vi "Autonomous Independent.vi"() -> ()   [LabVIEW 2011]
doc: "This VI is called when autonomous begins, and will automatically be terminated when autonomous ends. You can carry out timed or sensor driven robot movement independently without needing to return to the caller."
uses:
  AutoDriveType.ctl
  AutonomousType.ctl
  StateMachineType.ctl
  Robot Global Data.vi
  <vilib>/addons/control/pid/pid.llb/PID (DBL).vi
  <vilib>/Rock Robotics/WPI/RobotDrive/WPI_RobotDriveArcadeDrive_Standard(NoSaturation).vi
  BasketType.ctl
  <vilib>/addons/control/pid/NI_PID_pid.lvlib
panel:
  out "LaunchCounter 3":i32
  out "LaunchCounter 2":i32
  out "LaunchCounter":i32
  in  "AutoDrive":T1
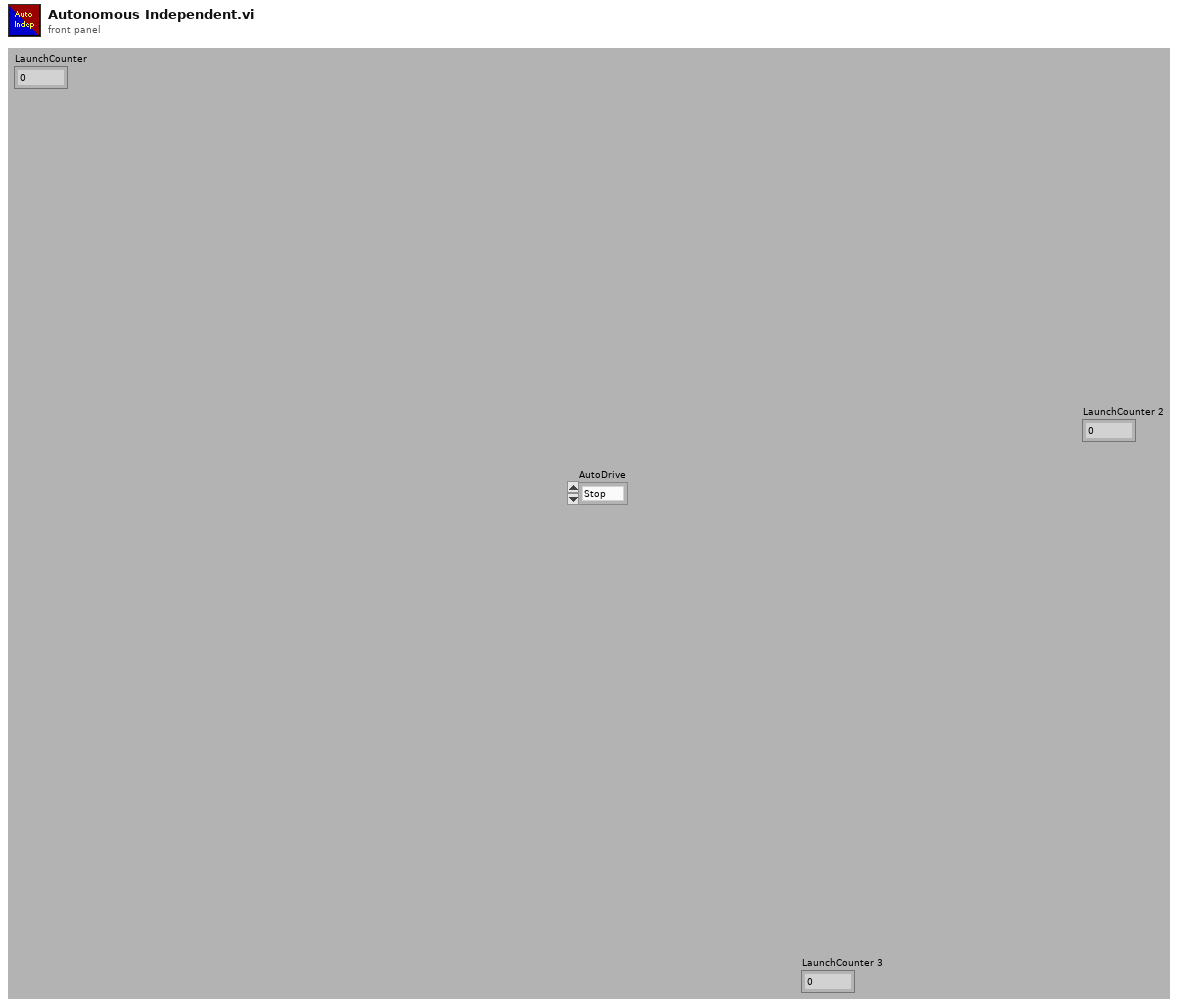
[diagram p1: front panel]
types:
  T1 = typedef "AutoDriveType.ctl" = enum16{"Stop", "DoNothing", "Drive"}
  T2 = typedef "WPI_RobotDriveDevRef.ctl" = cluster{"DevStatus":errorcluster, "Motors[]":T3[], "Square Inputs":bool, "Max Output":dbl, "Isochronous":bool}
  T3 = typedef "WPI_MotorControlDeviceRef.ctl" = cluster{"DeviceStatus":errorcluster, "Type":enum16{"PWM", "CAN"}, "PWM":cluster{"Digital Module":T4, "PWM Channel":T5, "DeadBand":T6}, "CAN":cluster{"Device Number":u8, "Control Mode":T7, "Semaphore":T8, "Max Vout":dbl}, "Invert":bool, "TransformRef":T9, "InvTransformRef":T9}
  T4 = typedef "FPGA_TypedefDigitalModule.ctl" = enum16{"Digital Module 1", "Digital Module 2"}
  T5 = typedef "FPGA_DIOPWMChannel.ctl" = enum8{"PWM 1", "PWM 2", "PWM 3", "PWM 4", "PWM 5", "PWM 6", "PWM 7", "PWM 8", "PWM 9", "PWM 10", "Invalid"}
  T6 = typedef "WPI_PWMDeadband.ctl" = cluster{"Name":string, "maxPositivePwm":i32, "minPositivePwm":i32, "centerPwm":i32, "maxNegativePwm":i32, "minNegativePwm":i32, "angularRange":u16}
  T7 = typedef "WPI_CANJaguar_ControlMode.ctl" = enum8{"Percent VBus", "Current", "Speed", "Position", "Voltage"}
  T8 = typedef "Semaphore RefNum" = refnum<k1>
  T9 = typedef "WPI_PWMTransform_ConPane.ctl" = refnum<vi>
  T10 = typedef "AutonomousType.ctl" = enum16{"Init", "ManualAim", "AutoAim", "Fire", "Drive", "Tip Ramp", "Stop"}
  T11 = typedef "BasketType.ctl" = enum16{"Left", "Bottom", "Right", "Top"}
  T12 = typedef "StateMachineType.ctl" = enum16{"Init", "Idle", "Start", "Do", "Stop"}
  T13 = cluster{"proportional gain (Kc)":dbl, "integral time (Ti, min)":dbl, "derivative time (Td, min)":dbl}
  T14 = cluster{"Position":cluster{"X":dbl, "Y":dbl}, "Distance (ft)":dbl}[]
  T15 = cluster{"Position":cluster{"X":dbl, "Y":dbl}, "Distance (ft)":dbl}
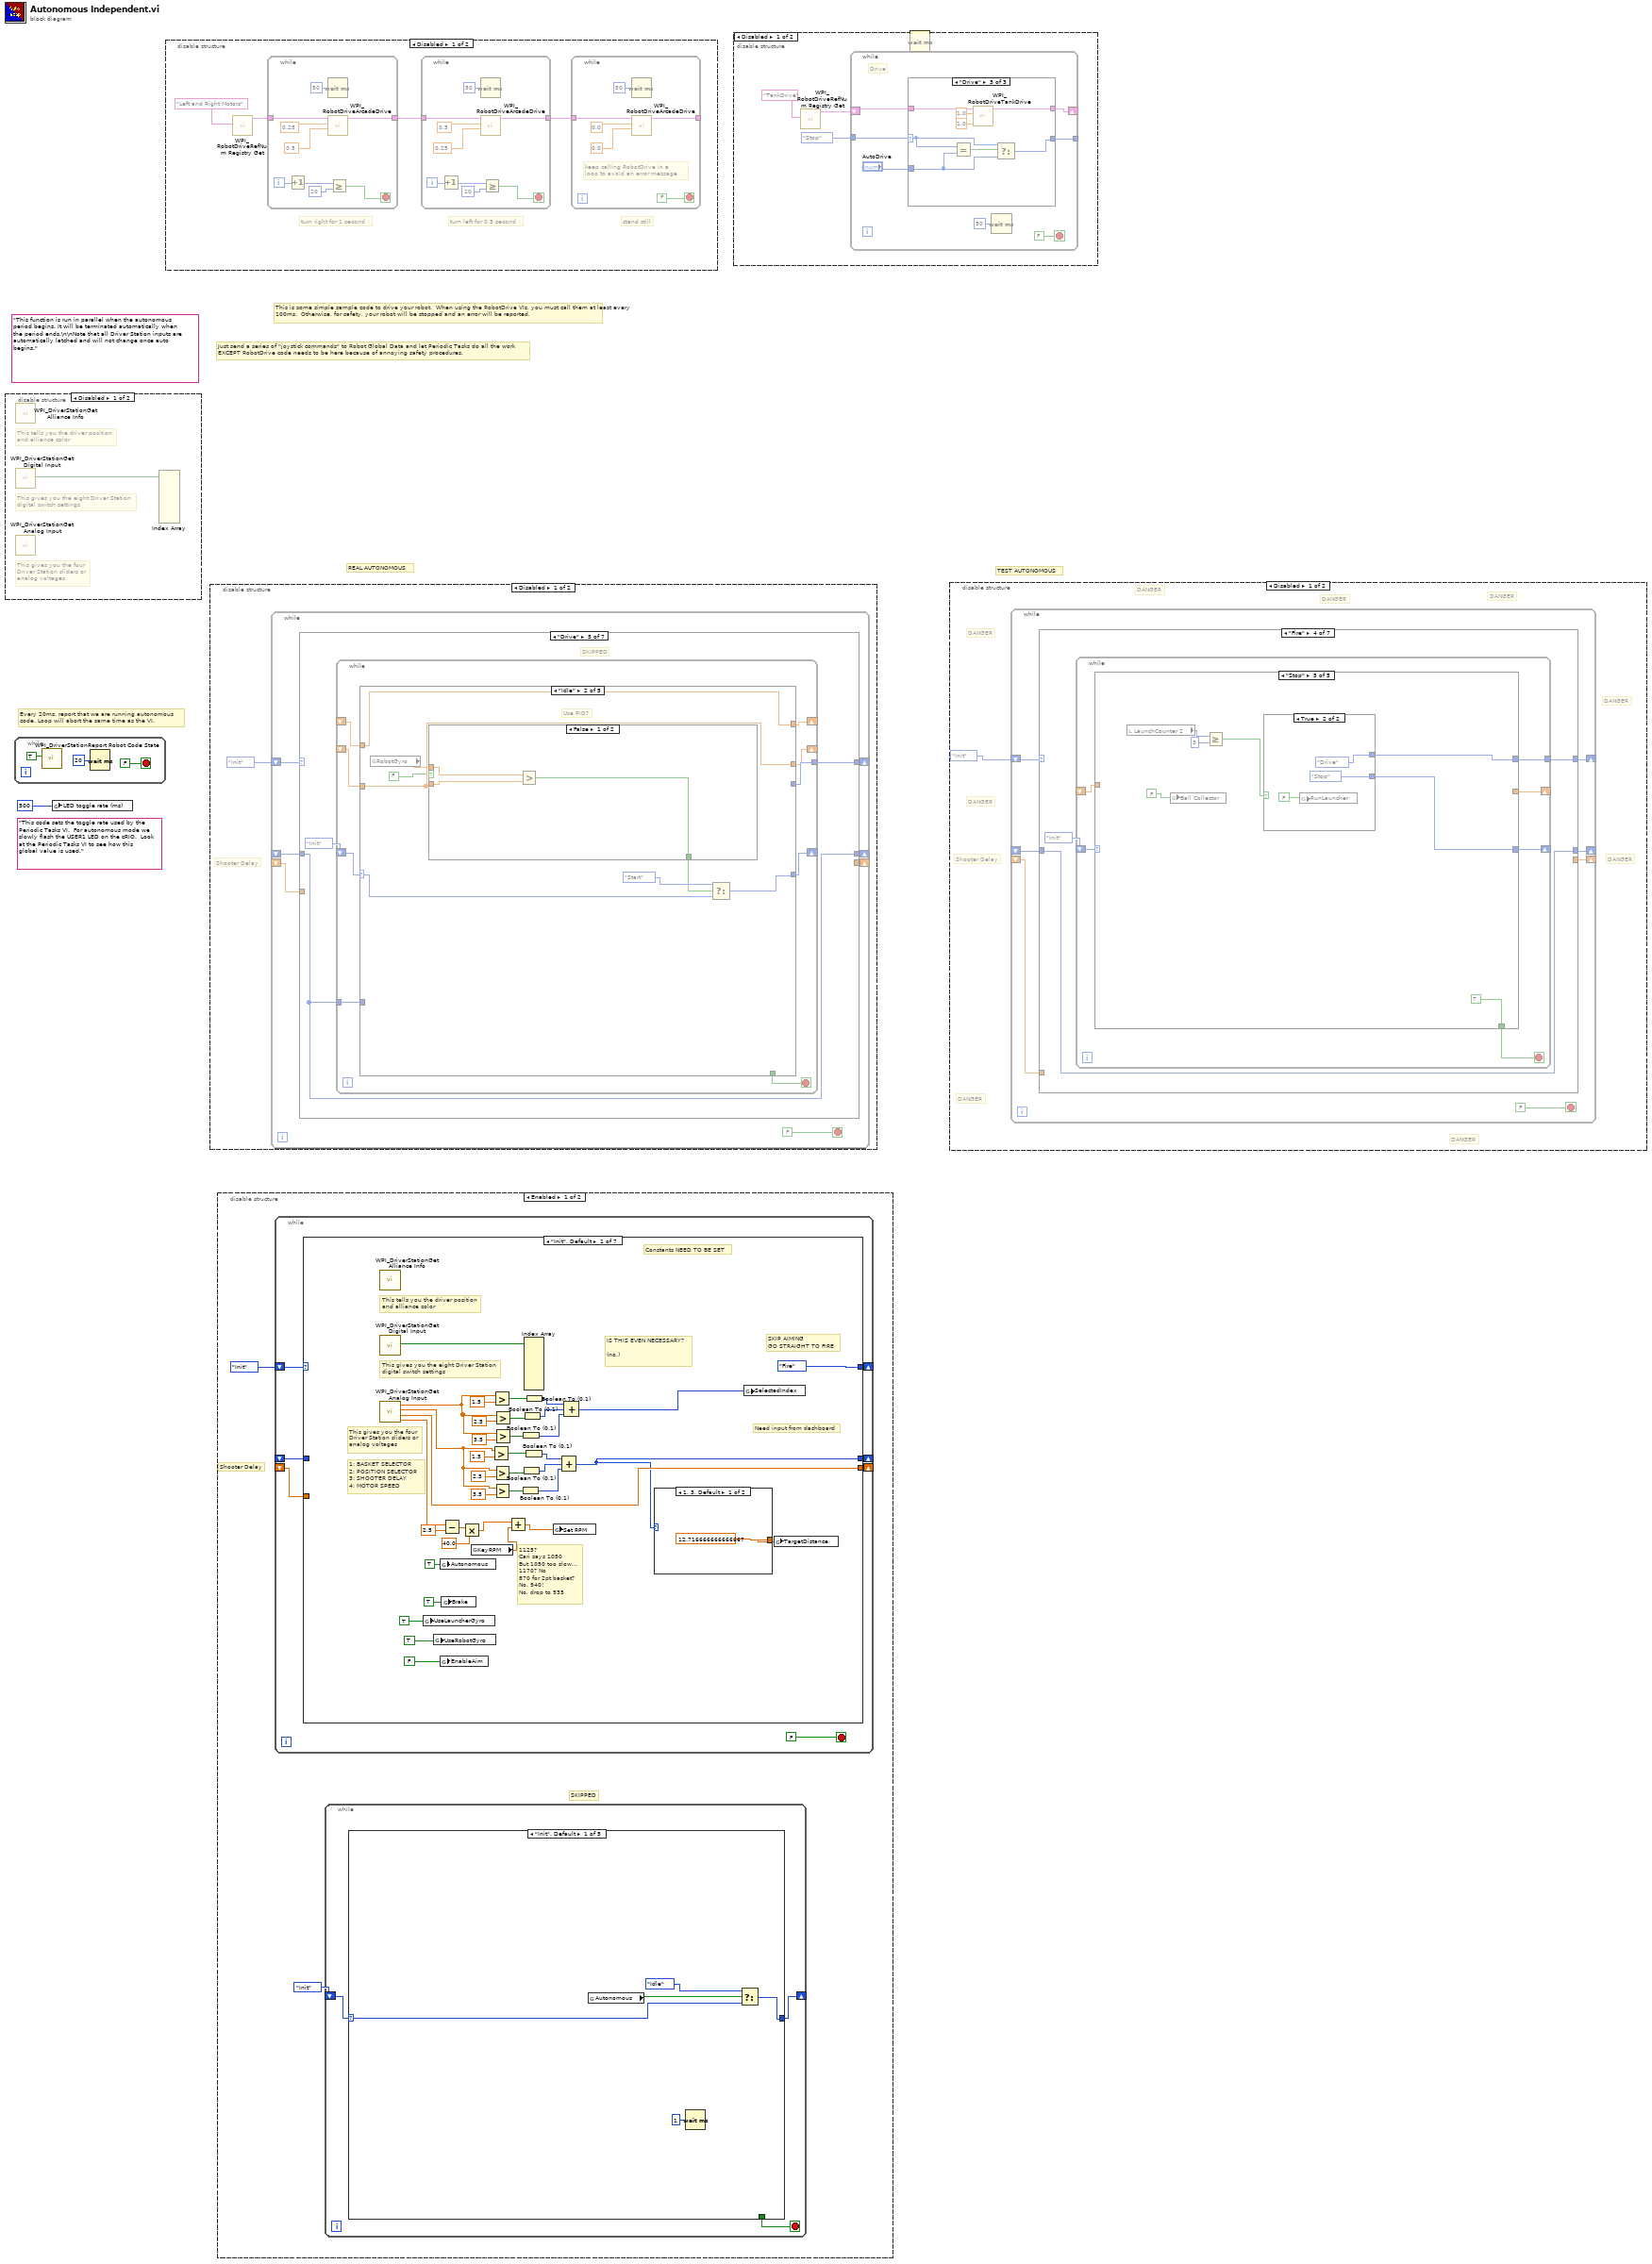
[diagram p0: block diagram]
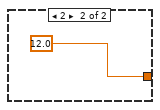
[diagram p2: hidden frame]
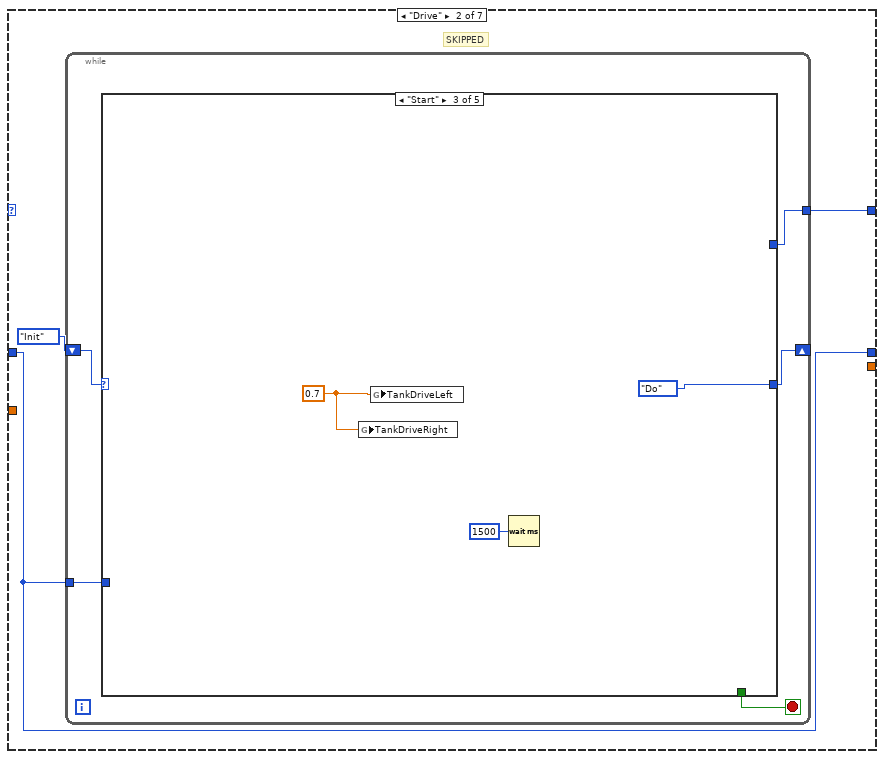
[diagram p3: hidden frame]
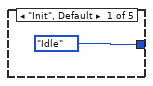
[diagram p4: hidden frame]
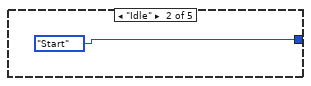
[diagram p5: hidden frame]
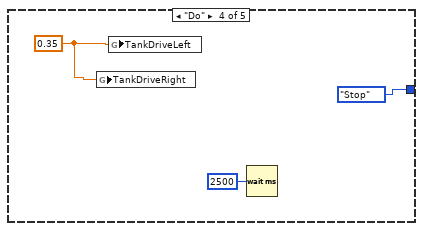
[diagram p6: hidden frame]
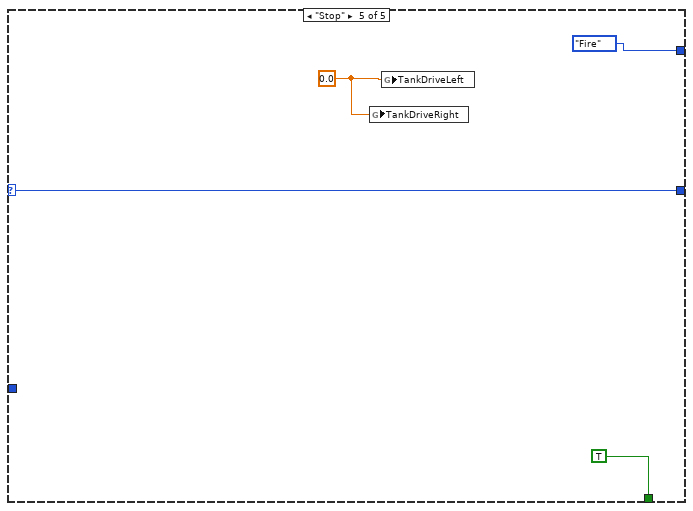
[diagram p7: hidden frame]
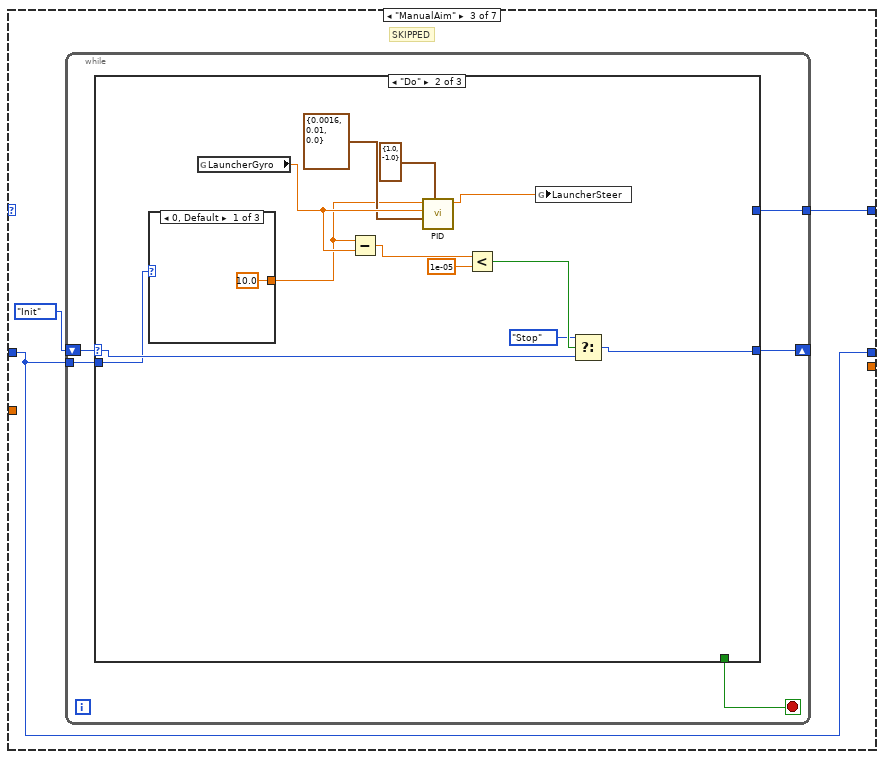
[diagram p8: hidden frame]
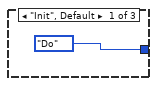
[diagram p9: hidden frame]
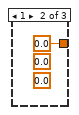
[diagram p10: hidden frame]
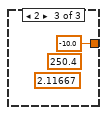
[diagram p11: hidden frame]
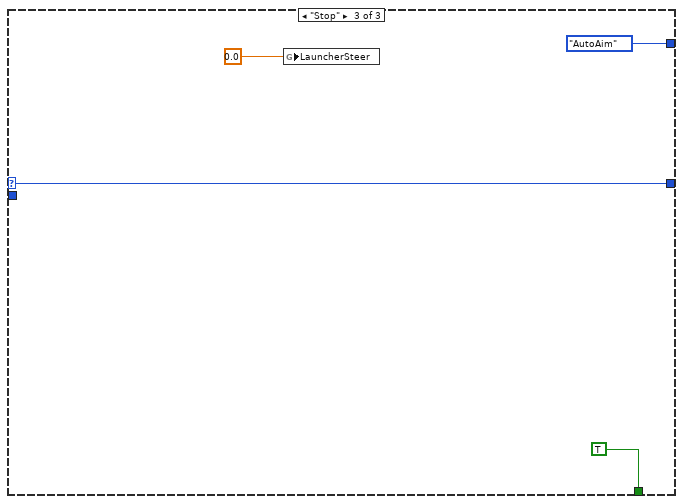
[diagram p12: hidden frame]
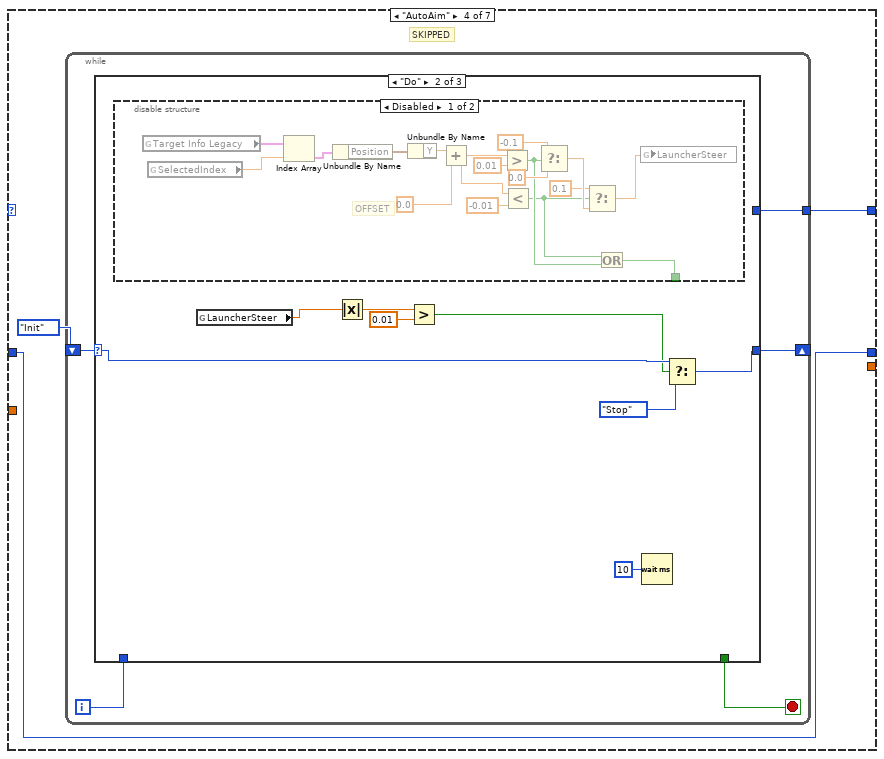
[diagram p13: hidden frame]
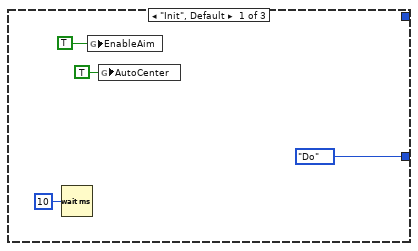
[diagram p14: hidden frame]
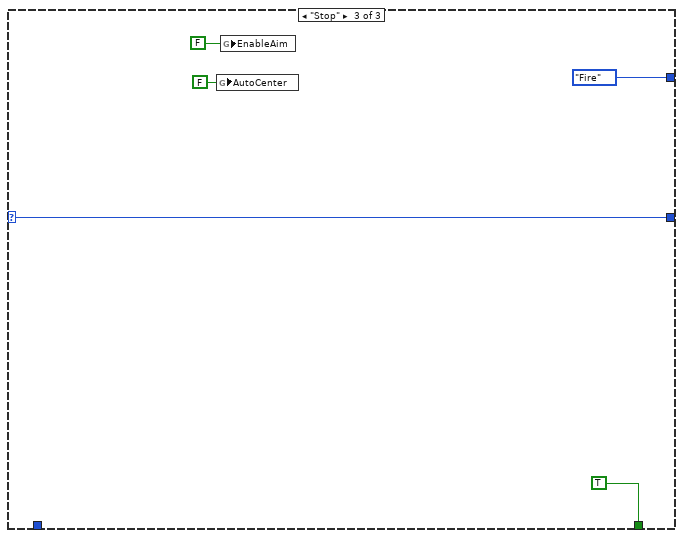
[diagram p16: hidden frame]
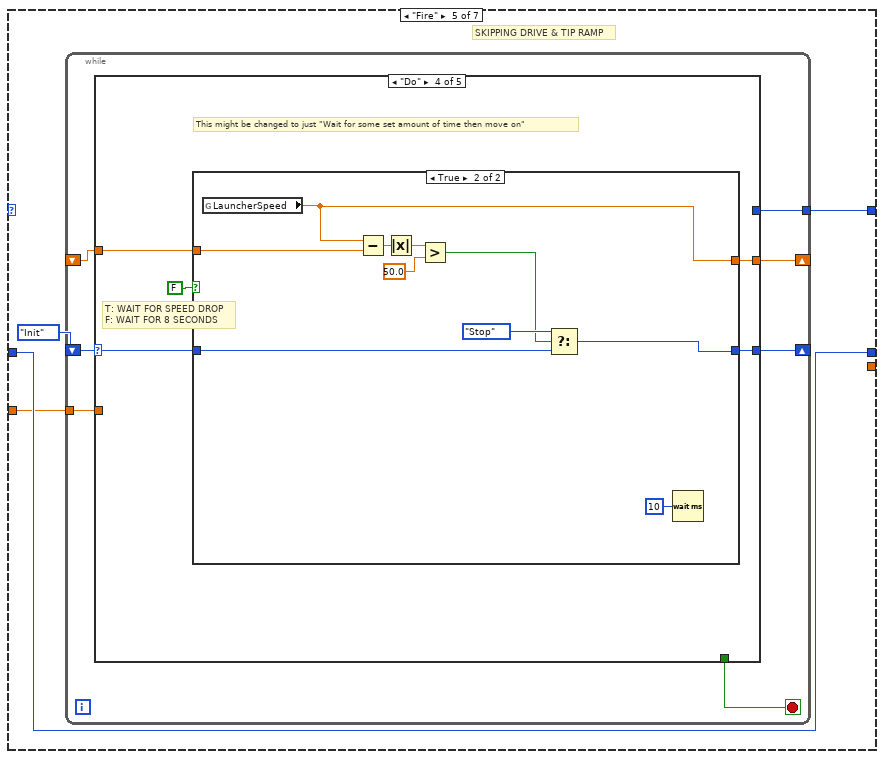
[diagram p17: hidden frame]
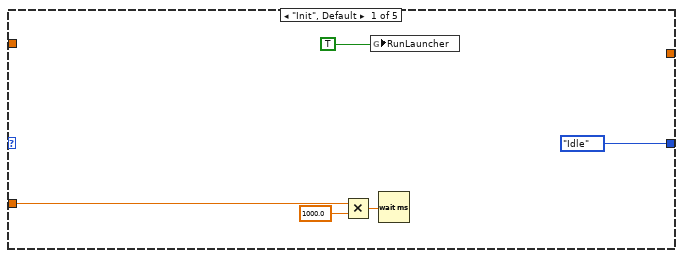
[diagram p18: hidden frame]
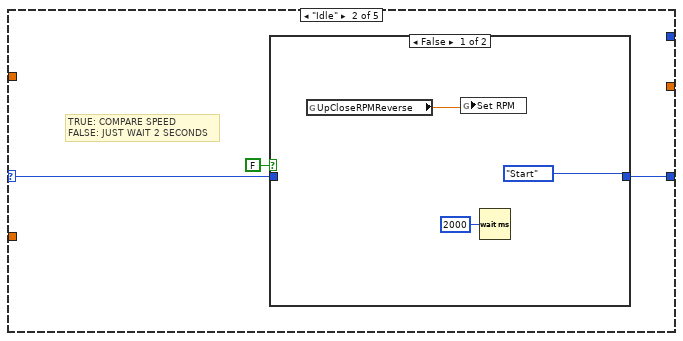
[diagram p19: hidden frame]
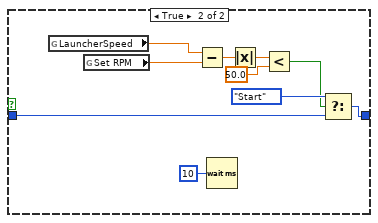
[diagram p20: hidden frame]
diagram:
  (unwired) "This code sets the toggle rate used by the Periodic Tasks VI.  For autonomous mode we slowly flash the USER1 LED on the cRIO.  Look at the Periodic Tasks VI to see how this global value is used."
  (unwired) "This function is run in parallel when the autonomous period begins. It will be terminated automatically when the period ends.\n\nNote that all Driver Station inputs are automatically latched and will not change once auto begins."
  # "TEST AUTONOMOUS"
  # "REAL AUTONOMOUS"
  # "This is some simple sample code to drive your robot.  When using the RobotDrive VIs, you must call them at least every 100ms.  Otherwise, for safety, your robot will be stopped and an error will be reported."
  # "Every 20ms, report that we are running autonomous\ncode. Loop will abort the same time as the VI."
  # "Just send a series of \"joystick commands\" to Robot Global Data and let Periodic Tasks do all the work\nEXCEPT RobotDrive code needs to be here because of annoying safety procedures."
  n1 = disable-structure shown="Disabled" {
    frame Disabled {
      # "This tells you the driver position\nand alliance color"
      # "This gives you the eight Driver Station\ndigital switch settings"
      # "This gives you the four\nDriver Station sliders or\nanalog voltages"
      n2 = call <vilib>:"WPI_DriverStationGet Alliance Info.vi"() -> ()  [unwired: 12 out]
      n3 = call <vilib>:"WPI_DriverStationGet Digital Input.vi"() -> ("Driver Station Digital Input (1-8)"=w2:bool[])  [unwired: 11 out]
      n4 = call <vilib>:"WPI_DriverStationGet Analog Input.vi"() -> ()  [unwired: 12 out]
      n5 = Index Array(array=w2) -> ()  [unwired: 8 in, 8 out]
    }
    frame Enabled {
    }
  }
  n6 = while {
    stop <- FALSE stop-if-true
    n7 = call <vilib>:"WPI_DriverStationReport Robot Code State.vi"("Autonomous"=TRUE) -> ()  [unwired: 10 in, 1 out]
    n8 = Wait (ms)(milliseconds to wait=u32 20) -> ()  [unwired: 1 out]
  }
  n9 = global write "Robot Global Data.vi" "LED toggle rate (ms)"(u32 500 ("LED ms toggle rate")) -> ()
  n10 = disable-structure shown="Disabled" {
    frame Disabled {
      # "stand still"
      # "turn left for 0.5 second"
      # "turn right for 1 second"
      n11 = call <vilib>:"WPI_RobotDriveRefNum Registry Get.vi"("refnum name"="Left and Right Motors") -> ("RobotDriveDevRef"=w8:T2)  [unwired: 1 in, 9 out]
      n12 = while {
        tunnel: w8 -> [w33]
        tunnel: [w26] -> w7
        i -> [w29]
        stop <- w27 stop-if-true
        n13 = Increment(x=w29) -> (x+1=w25:i32)
        n14 = Wait (ms)(milliseconds to wait=u32 50) -> ()  [unwired: 1 out]
        n15 = call-poly <vilib>:"WPI_RobotDriveArcadeDrive.vi"("Y axis value"=0.5 ("X axis value"), "X axis value"=0.25, "RobotDriveDevRef"=w33) -> ("RobotDriveDevRef"=w26:T2)  [unwired: 1 in, 7 out]
        n16 = Greater Or Equal?(x=w25, y=20) -> (x >= y?=w27:bool)
      }
      n17 = while {
        tunnel: w7 -> [w24]
        tunnel: [w17] -> w6
        i -> [w20]
        stop <- w18 stop-if-true
        n18 = Increment(x=w20) -> (x+1=w16:i32)
        n19 = Wait (ms)(milliseconds to wait=u32 50) -> ()  [unwired: 1 out]
        n20 = call-poly <vilib>:"WPI_RobotDriveArcadeDrive.vi"("Y axis value"=0.25 ("X axis value"), "X axis value"=0.5, "RobotDriveDevRef"=w24) -> ("RobotDriveDevRef"=w17:T2)  [unwired: 1 in, 7 out]
        n21 = Greater Or Equal?(x=w16, y=10) -> (x >= y?=w18:bool)
      }
      n22 = while {
        tunnel: w6 -> [w15]
        tunnel: [w11] -> _
        stop <- FALSE stop-if-true
        # "keep calling RobotDrive in a loop to avoid an error message"
        n23 = Wait (ms)(milliseconds to wait=u32 50) -> ()  [unwired: 1 out]
        n24 = call-poly <vilib>:"WPI_RobotDriveArcadeDrive.vi"("Y axis value"=0.0 ("X axis value"), "X axis value"=0.0, "RobotDriveDevRef"=w15) -> ("RobotDriveDevRef"=w11:T2)  [unwired: 1 in, 7 out]
      }
    }
    frame Enabled {
    }
  }
  n25 = disable-structure shown="Disabled" {
    frame Disabled {
      # "Shooter Delay"
      n26 = while {
        shift-right: [w40] -> _
        shift-left: _ -> [w35]
        shift-right: [w38] -> _
        shift-left: AutonomousType."Init" -> [w41]
        shift-right: [w37] -> _
        shift-left: _ -> [w36]
        stop <- FALSE stop-if-true
        n27 = case shown="\"Drive\"" w41 {
          selector: w41 -> [_ _ _ _ _ _ w330]
          tunnel: [w54 _ _ _ _ _ _] -> w40
          tunnel: [AutonomousType."Fire" ("Enum") w87 w115 w150 w218 w298 w330] -> w38
          tunnel: [w51 w86 w114 w149 w217 _ _] -> w37
          tunnel: w36 -> [_ w86 w114 w149 w217 _ _]
          tunnel: w35 -> [_ _ _ w148 _ _ _]
          frame "Init", Default {
            # "1125?\nCari says 1050 \nBut 1050 too slow...\n1170? No\n870 for 2pt basket?\nNo. 940!\nNo, drop to 935"
            # "IS THIS EVEN NECESSARY?"
            # "SKIP AIMING\nGO STRAIGHT TO FIRE"
            # "Need input from dashboard"
            # "1: BASKET SELECTOR\n2: POSITION SELECTOR\n3: SHOOTER DELAY\n4: MOTOR SPEED"
            # "Constants NEED TO BE SET"
            # "This tells you the driver position\nand alliance color"
            # "This gives you the eight Driver Station\ndigital switch settings"
            # "This gives you the four\nDriver Station sliders or\nanalog voltages"
            n28 = call <vilib>:"WPI_DriverStationGet Alliance Info.vi"() -> ()  [unwired: 12 out]
            n29 = call <vilib>:"WPI_DriverStationGet Digital Input.vi"() -> ("Driver Station Digital Input (1-8)"=w79:bool[])  [unwired: 11 out]
            n30 = call <vilib>:"WPI_DriverStationGet Analog Input.vi"() -> ("Analog 4 (V)"=w48:dbl, "Analog 3 (V)"=w54:dbl, "Analog 2 (V)"=w55:dbl, "Analog 1 (V)"=w67:dbl)  [unwired: 8 out]
            n31 = global write "Robot Global Data.vi" "UseLauncherGyro"(TRUE) -> ()
            n32 = global write "Robot Global Data.vi" "UseRobotGyro"(TRUE) -> ()
            n33 = global write "Robot Global Data.vi" "Autonomous"(TRUE ("Autonomous")) -> ()
            n34 = global write "Robot Global Data.vi" "Brake"(TRUE) -> ()
            n35 = Subtract(x=w48, y=2.5) -> (x-y=w46:dbl)
            n36 = Multiply(x=w46, y=40.0) -> (x*y=w43:dbl)
            n37 = global read "Robot Global Data.vi" "KeyRPM"() -> (w42:dbl)
            n38 = Greater?(x=w55, y=1.5) -> (0:w59:bool)
            n39 = Greater?(x=w67, y=1.5) -> (0:w73:bool)
            n40 = Greater?(x=w55, y=2.5) -> (0:w60:bool)
            n41 = Greater?(x=w55, y=3.5) -> (0:w61:bool)
            n42 = Greater?(x=w67, y=2.5) -> (0:w74:bool)
            n43 = Greater?(x=w67, y=3.5) -> (0:w75:bool)
            n44 = Add(x=w43, y=w42) -> (x+y=w44:dbl)
            n45 = Boolean To (0,1)(Boolean=w61) -> (0, 1=w56:i16)
            n46 = Boolean To (0,1)(Boolean=w75) -> (0, 1=w70:i16)
            n47 = Boolean To (0,1)(Boolean=w60) -> (0, 1=w57:i16)
            n48 = Boolean To (0,1)(Boolean=w74) -> (0, 1=w71:i16)
            n49 = Boolean To (0,1)(Boolean=w59) -> (0, 1=w58:i16)
            n50 = Index Array(array=w79) -> ()  [unwired: 8 in, 8 out]
            n51 = Boolean To (0,1)(Boolean=w73) -> (0, 1=w72:i16)
            n52 = global write "Robot Global Data.vi" "Set RPM"(w44) -> ()
            n53 = Compound Arithmetic op=ADD(w58, w57, w56) -> (w51:i16)
            n54 = Compound Arithmetic op=ADD(w72, w71, w70) -> (w69:i16)
            n55 = case shown="0, Default" w69 {
              tunnel: [BasketType."Left" ("Basket") BasketType."Bottom" ("Basket") BasketType."Right" ("Basket") BasketType."Top" ("Basket")] -> w68
              frame 0, Default {
              }
              frame 1 {
              }
              frame 2 {
              }
              frame 3 {
              }
            }
            n56 = case shown="1, 3, Default" w51 {
              tunnel: [12.716666666666667 12.0] -> w52
              frame 1, 3, Default {
              }
              frame 2 {
              }
            }
            n57 = global write "Robot Global Data.vi" "Basket"(w68) -> ()
            n58 = global write "Robot Global Data.vi" "TargetDistance"(w52) -> ()
          }
          frame "ManualAim" {
            # "SKIPPED"
            n59 = while {
              shift-right: [w92] -> _
              shift-left: StateMachineType."Init" ("Enum") -> [w93]
              tunnel: [w90] -> w87
              tunnel: w86 -> [w89]
              stop <- w91 stop-if-true
              n60 = case shown="\"Do\"" w93 {
                selector: w93 -> [_ w100 w112]
                tunnel: [StateMachineType."Do" ("Enum") w99 w112] -> w92
                tunnel: [_ _ TRUE] -> w91
                tunnel: [_ _ AutonomousType."AutoAim" ("Enum")] -> w90
                tunnel: w89 -> [_ w95 _]
                frame "Init", Default {
                }
                frame "Do" {
                  n61 = case shown="0, Default" w95 {
                    tunnel: [10.0 0.0 -10.0] -> w96
                    frame 0, Default {
                    }
                    frame 1 {
                      (unwired) 0.0
                      (unwired) 0.0
                    }
                    frame 2 {
                      (unwired) 2.11667
                      (unwired) 250.4
                    }
                  }
                  n62 = global read "Robot Global Data.vi" "LauncherGyro"() -> (w104:dbl)
                  n63 = Subtract(x=w96, y=w104) -> (x-y=w103:dbl)
                  n64 = call-poly <vilib>:"PID.vi"("output range"=cluster{"output high":dbl, "output low":dbl} {"output high"=1.0, "output low"=-1.0}, "PID gains"=T13 {"proportional gain (Kc)"=0.0016, "integral time (Ti, min)"=0.01, "derivative time (Td, min)"=0.0}, "process variable"=w104, "setpoint"=w96) -> ("output"=w105:dbl)  [unwired: 6 in, 1 out]
                  n65 = Less?(x=w103, y=1e-05) -> (x < y?=w101:bool)
                  n66 = global write "Robot Global Data.vi" "LauncherSteer"(w105) -> ()
                  n67 = Select(t=StateMachineType."Stop", s=w101, f=w100) -> (s? t:f=w99:T12)
                }
                frame "Stop" {
                  n68 = global write "Robot Global Data.vi" "LauncherSteer"(0.0 ("LauncherSteer")) -> ()
                }
              }
            }
          }
          frame "AutoAim" {
            # "SKIPPED"
            n69 = while {
              shift-right: [w120] -> _
              shift-left: StateMachineType."Init" ("Enum") -> [w121]
              tunnel: [w117] -> w115
              i -> [w118]
              stop <- w119 stop-if-true
              n70 = case shown="\"Init\", Default" w121 {
                selector: w121 -> [_ w128 w146]
                tunnel: [StateMachineType."Do" ("Enum") w127 w146] -> w120
                tunnel: [_ _ TRUE] -> w119
                tunnel: w118 -> [_ _ _]
                tunnel: [_ _ AutonomousType."Fire" ("Enum")] -> w117
                frame "Init", Default {
                  n71 = global write "Robot Global Data.vi" "EnableAim"(TRUE ("Enable Vision")) -> ()
                }
                frame "Do" {
                  n72 = global read "Robot Global Data.vi" "Target Info Legacy"() -> (w143:T14)
                  n73 = global read "Robot Global Data.vi" "SelectedIndex"() -> (w142:dbl)
                  n74 = Index Array(array=w143, index=w142) -> (element=w141:T15)
                  n75 = Unbundle By Name(w141) -> ("Position"=w140:cluster{"X":dbl, "Y":dbl})
                  n76 = Unbundle By Name(w140) -> ("Y"=w139:dbl)
                  n77 = Add(x=w139, y=0.0) -> (x+y=w124:dbl)
                  n78 = Greater?(x=w124, y=0.01) -> (0:w131:bool)
                  n79 = Less?(x=w124, y=-0.01) -> (x < y?=w130:bool)
                  n80 = Select(t=-0.1, s=w131, f=0.0) -> (s? t:f=w134:dbl)
                  n81 = Select(t=0.1, s=w130, f=w134) -> (s? t:f=w132:dbl)
                  n82 = Or(x=w130, y=w131) -> (x .or. y?=w129:bool)
                  n83 = global write "Robot Global Data.vi" "LauncherSteer"(w132) -> ()
                  n84 = Select(t=w128, s=w129, f=StateMachineType."Stop") -> (s? t:f=w127:T12)
                }
                frame "Stop" {
                  n85 = global write "Robot Global Data.vi" "EnableAim"(FALSE ("Enable Vision")) -> ()
                }
              }
            }
          }
          frame "Fire" {
            # "SKIPPING DRIVE & TIP RAMP"
            n86 = while {
              shift-right: [w157] -> _
              shift-left: StateMachineType."Init" ("Enum") -> [w158]
              tunnel: [w155] -> w150
              shift-right: [w154] -> _
              shift-left: _ -> [w153]
              tunnel: w148 -> [w152]
              stop <- w156 stop-if-true
              n87 = case shown="\"Idle\"" w158 {
                selector: w158 -> [_ w165 _ w186 _]
                tunnel: [StateMachineType."Idle" ("Enum") w166 StateMachineType."Do" ("Enum") w185 w208] -> w157
                tunnel: [_ _ _ _ TRUE] -> w156
                tunnel: [_ _ _ _ w209] -> w155
                tunnel: [_ _ _ w188 _] -> w154
                tunnel: w153 -> [_ _ _ w187 _]
                tunnel: w152 -> [w160 _ _ _ _]
                frame "Init", Default {
                  n88 = Multiply(x=w160, y=1000.0) -> (x*y=w161:dbl)
                  n89 = global write "Robot Global Data.vi" "RunLauncher"(TRUE) -> ()
                  n90 = Wait (ms)(milliseconds to wait=w161) -> ()  [unwired: 1 out]
                }
                frame "Idle" {
                  # "TRUE: COMPARE SPEED\nFALSE: JUST WAIT 2 SECONDS"
                  n91 = case shown="False" FALSE {
                    tunnel: [StateMachineType."Start" ("Enum") w171] -> w166
                    tunnel: w165 -> [_ w169]
                    frame False {
                      n92 = Wait (ms)(milliseconds to wait=u32 2000) -> ()  [unwired: 1 out]
                    }
                    frame True {
                      n93 = global read "Robot Global Data.vi" "LauncherSpeed"() -> (w176:dbl)
                      n94 = global read "Robot Global Data.vi" "Set RPM"() -> (w175:dbl)
                      n95 = Subtract(x=w176, y=w175) -> (x-y=w174:dbl)
                      n96 = Wait (ms)(milliseconds to wait=u32 10) -> ()  [unwired: 1 out]
                      n97 = Absolute Value(x=w174) -> (abs(x)=w172:dbl)
                      n98 = Less?(x=w172, y=50.0) -> (x < y?=w170:bool)
                      n99 = Select(t=StateMachineType."Start" ("Enum"), s=w170, f=w169) -> (s? t:f=w171:T12)
                    }
                  }
                }
                frame "Start" {
                  # "IN PERIODIC TASKS CREATE A BOOLEAN\nCONFIRMING THAT LAUNCHER IS UP TO SPEED"
                  # "MAKE FOR LOOP"
                  n100 = local read "LaunchCounter"() -> (w181:i32)
                  n101 = global write "Robot Global Data.vi" "Ball Collector"(TRUE) -> ()
                  n102 = global write "Robot Global Data.vi" "Fire"(TRUE) -> ()
                  n103 = Increment(x=w181) -> (x+1=→"LaunchCounter":i32)
                }
                frame "Do" {
                  # "T: WAIT FOR SPEED DROP\nF: WAIT FOR 8 SECONDS"
                  # "This might be changed to just \"Wait for some set amount of time then move on\""
                  n104 = case shown="False" FALSE {
                    tunnel: [w191 w201] -> w188
                    tunnel: w187 -> [w191 w200]
                    tunnel: w186 -> [_ w195]
                    tunnel: [StateMachineType."Stop" ("t") w193] -> w185
                    frame False {
                      n105 = Wait (ms)(milliseconds to wait=u32 8000) -> ()  [unwired: 1 out]
                    }
                    frame True {
                      n106 = global read "Robot Global Data.vi" "LauncherSpeed"() -> (w201:dbl)
                      n107 = Subtract(x=w201, y=w200) -> (x-y=w199:dbl)
                      n108 = Absolute Value(x=w199) -> (abs(x)=w197:dbl)
                      n109 = Greater?(x=w197, y=50.0) -> (0:w194:bool)
                      n110 = Select(t=StateMachineType."Stop", s=w194, f=w195) -> (s? t:f=w193:T12)
                      n111 = Wait (ms)(milliseconds to wait=u32 10) -> ()  [unwired: 1 out]
                    }
                  }
                }
                frame "Stop" {
                  # "T: WAIT FOR 2 BALLS LAUNCHED\nF: JUST STOP"
                  # "# OF BALLS IN COLLECTOR"
                  # "SKIPPING DRIVE"
                  n112 = global write "Robot Global Data.vi" "Ball Collector"(FALSE) -> ()
                  n113 = local read "LaunchCounter"() -> (w211:i32)
                  n114 = global write "Robot Global Data.vi" "Fire"(FALSE) -> ()
                  n115 = Select(t=2, s=FALSE, f=0 ("y")) -> (s? t:f=w202:i32)
                  n116 = Greater Or Equal?(x=w211, y=w202) -> (x >= y?=w210:bool)
                  n117 = case shown="True" w210 {
                    tunnel: [_ AutonomousType."Stop" ("Enum")] -> w209
                    tunnel: [StateMachineType."Idle" ("Enum") StateMachineType."Stop" ("Enum")] -> w208
                    frame False {
                    }
                    frame True {
                      # "SKIPPING DRIVE & TIP RAMP"
                      n118 = global write "Robot Global Data.vi" "RunLauncher"(FALSE) -> ()
                    }
                  }
                }
              }
            }
          }
          frame "Drive" {
            # "SKIPPED"
            n119 = while {
              shift-right: [w227] -> _
              shift-left: StateMachineType."Init" ("Enum") -> [w228]
              tunnel: [w225] -> w218
              shift-right: [w221] -> _
              shift-left: _ -> [w224]
              shift-right: [w223] -> _
              shift-left: _ -> [w222]
              tunnel: w217 -> [w220]
              stop <- w226 stop-if-true
              n120 = case shown="\"Idle\"" w228 {
                selector: w228 -> [_ w263 _ w288 w296]
                tunnel: [StateMachineType."Idle" ("Enum") w264 StateMachineType."Do" ("Enum") w287 w296] -> w227
                tunnel: [_ _ _ _ TRUE] -> w226
                tunnel: [_ _ _ _ AutonomousType."Tip Ramp" ("Enum")] -> w225
                tunnel: w224 -> [_ w261 w280 w285 _]
                tunnel: w222 -> [_ w266 _ _ _]
                tunnel: [w233 w266 _ _ _] -> w223
                tunnel: [w234 w261 w280 w285 _] -> w221
                tunnel: w220 -> [w235 _ _ _ _]
                frame "Init", Default {
                  # "BRIDGE Y COORDINATE"
                  # "DESIRED DISTANCE"
                  # "BRIDGE X COORDINATE"
                  # "DESIRED ANGLE"
                  n121 = global read "Robot Global Data.vi" "LauncherGyro"() -> (w237:dbl)
                  n122 = global read "Robot Global Data.vi" "TargetDistance"() -> (w238:dbl)
                  n123 = case shown="1, Default" w235 {
                    tunnel: [7.05 0.0 -7.05] -> w239
                    frame 1, Default {
                    }
                    frame 2 {
                    }
                    frame 3 {
                    }
                  }
                  n124 = Multiply(x=w237, y=3.141592653589793) -> (x*y=w232:dbl)
                  n125 = Divide(x=w232, y=180.0) -> (x/y=w231:dbl)
                  n126 = Sine & Cosine(0:w231) -> (1:w249:dbl, 2:w248:dbl)
                  n127 = Multiply(x=w248, y=w238) -> (x*y=w254:dbl)
                  n128 = Multiply(x=w249, y=w238) -> (x*y=w255:dbl)
                  n129 = Add(x=w239, y=w255) -> (x+y=w246:dbl)
                  n130 = Subtract(x=20.8666667, y=w254) -> (x-y=w247:dbl)
                  n131 = Square(x=w247) -> (x^2=w252:dbl)
                  n132 = Square(x=w246) -> (x^2=w251:dbl)
                  n133 = Add(x=w252, y=w251) -> (x+y=w250:dbl)
                  n134 = Square Root(x=w250) -> (sqrt(x)=w234:dbl)
                  n135 = Inverse Tangent (2 Input)(1:w246, 2:w247) -> (0:w244:dbl)
                  n136 = Add(x=1.5707963267948966, y=w244) -> (x+y=w242:dbl)
                  n137 = Divide(x=w242, y=3.141592653589793) -> (x/y=w241:dbl)
                  n138 = Multiply(x=180.0, y=w241) -> (x*y=w233:dbl)
                }
                frame "Idle" {
                  # "Use PID?"
                  n139 = global read "Robot Global Data.vi" "RobotGyro"() -> (w259:dbl)
                  n140 = case shown="False" FALSE {
                    tunnel: w266 -> [w268 w272]
                    tunnel: [w267 w271] -> w262
                    tunnel: w259 -> [w269 w270]
                    frame False {
                      n141 = Greater?(x=w269, y=w268) -> (0:w267:bool)
                    }
                    frame True {
                      n142 = Subtract(x=w270, y=w272) -> (x-y=w275:dbl)
                      n143 = call-poly <vilib>:"PID.vi"("output range"=cluster{"output high":dbl, "output low":dbl} {"output high"=1.0, "output low"=-1.0}, "PID gains"=T13 {"proportional gain (Kc)"=0.0016, "integral time (Ti, min)"=0.01, "derivative time (Td, min)"=0.0}, "process variable"=w270, "setpoint"=w272) -> ("output"=w278:dbl)  [unwired: 6 in, 1 out]
                      n144 = Absolute Value(x=w275) -> (abs(x)=w274:dbl)
                      n145 = Negate(x=w278) -> (-x=w277:dbl)
                      n146 = global write "Robot Global Data.vi" "TankDriveRight"(w277) -> ()
                      n147 = global write "Robot Global Data.vi" "TankDriveLeft"(w278) -> ()
                      n148 = Less?(x=w274, y=1.0) -> (x < y?=w271:bool)
                    }
                  }
                  n149 = Select(t=StateMachineType."Start" ("Enum"), s=w262, f=w263) -> (s? t:f=w264:T12)
                }
                frame "Start" {
                  # "Start driving straight"
                  n150 = global write "Robot Global Data.vi" "ReadDriveEncoders"(TRUE) -> ()
                  n151 = global write "Robot Global Data.vi" "TankDriveLeft"(1.0 ("TankDriveLeft")) -> ()
                  n152 = global write "Robot Global Data.vi" "StraightDrive"(TRUE) -> ()
                }
                frame "Do" {
                  n153 = global read "Robot Global Data.vi" "DriveDistance"() -> (w290:dbl)
                  n154 = Greater?(x=w290, y=w285) -> (0:w286:bool)
                  n155 = case shown="True" w286 {
                    frame False {
                    }
                    frame True {
                      n156 = Wait (ms)(milliseconds to wait=u32 50) -> ()  [unwired: 1 out]
                    }
                  }
                  n157 = Select(t=StateMachineType."Stop", s=w286, f=w288) -> (s? t:f=w287:T12)
                }
                frame "Stop" {
                  n158 = global write "Robot Global Data.vi" "ReadDriveEncoders"(FALSE) -> ()
                  n159 = global write "Robot Global Data.vi" "TankDriveLeft"(0.0 ("TankDriveLeft")) -> ()
                  n160 = global write "Robot Global Data.vi" "StraightDrive"(FALSE) -> ()
                }
              }
            }
          }
          frame "Tip Ramp" {
            # "SKIPPED"
            n161 = while {
              shift-right: [w302] -> _
              shift-left: StateMachineType."Init" ("Enum") -> [w303]
              tunnel: [w300] -> w298
              stop <- w301 stop-if-true
              n162 = case shown="\"Idle\"" w303 {
                selector: w303 -> [_ w312 _ _ w324]
                tunnel: [StateMachineType."Idle" ("Enum") w311 StateMachineType."Do" ("Enum") StateMachineType."Stop" ("t") w324] -> w302
                tunnel: [_ _ _ _ TRUE] -> w301
                tunnel: [_ _ _ _ AutonomousType."Stop" ("Enum")] -> w300
                frame "Init", Default {
                }
                frame "Idle" {
                  w309 = 180.0 ("setpoint")
                  # "USE PID TO FACE RAMP"
                  n163 = global read "Robot Global Data.vi" "RobotGyro"() -> (w310:dbl)
                  n164 = Subtract(x=w310, y=w309) -> (x-y=w308:dbl)
                  n165 = call-poly <vilib>:"PID.vi"("output range"=cluster{"output high":dbl, "output low":dbl} {"output high"=1.0, "output low"=-1.0}, "PID gains"=T13 {"proportional gain (Kc)"=0.0016, "integral time (Ti, min)"=0.01, "derivative time (Td, min)"=0.0}, "process variable"=w310, "setpoint"=w309) -> ("output"=w316:dbl)  [unwired: 6 in, 1 out]
                  n166 = Absolute Value(x=w308) -> (abs(x)=w307:dbl)
                  n167 = Negate(x=w316) -> (-x=w315:dbl)
                  n168 = global write "Robot Global Data.vi" "TankDriveRight"(w315) -> ()
                  n169 = global write "Robot Global Data.vi" "TankDriveLeft"(w316) -> ()
                  n170 = Less?(x=w307, y=1.0) -> (x < y?=w305:bool)
                  n171 = Select(t=StateMachineType."Start" ("Enum"), s=w305, f=w312) -> (s? t:f=w311:T12)
                }
                frame "Start" {
                  n172 = global write "Robot Global Data.vi" "ArmActuate"(TRUE ("Arm")) -> ()
                }
                frame "Do" {
                  n173 = Wait (ms)(milliseconds to wait=u32 1000) -> ()  [unwired: 1 out]
                }
                frame "Stop" {
                  n174 = global write "Robot Global Data.vi" "ArmActuate"(FALSE) -> ()
                }
              }
            }
          }
          frame "Stop" {
            # "YAY DONE"
            n175 = global write "Robot Global Data.vi" "Autonomous"(FALSE) -> ()
            n176 = global write "Robot Global Data.vi" "UseLauncherGyro"(FALSE) -> ()
            n177 = global write "Robot Global Data.vi" "UseRobotGyro"(FALSE) -> ()
            n178 = Wait (ms)(milliseconds to wait=u32 100) -> ()  [unwired: 1 out]
          }
        }
      }
    }
    frame Enabled {
    }
  }
  n179 = disable-structure shown="Enabled" {
    frame Enabled {
      # "Shooter Delay"
      # "SKIPPED"
      n180 = while {
        shift-right: [w338] -> _
        shift-left: _ -> [w333]
        shift-right: [w336] -> _
        shift-left: AutonomousType."Init" -> [w339]
        shift-right: [w335] -> _
        shift-left: _ -> [w334]
        stop <- FALSE stop-if-true
        n181 = case shown="\"Init\", Default" w339 {
          selector: w339 -> [_ _ _ _ _ _ w574]
          tunnel: [w354 _ _ _ _ _ _] -> w338
          tunnel: [AutonomousType."Fire" ("Enum") w381 w401 w429 w472 w542 w574] -> w336
          tunnel: [w351 w380 w400 w428 w471 _ _] -> w335
          tunnel: w334 -> [_ w380 w400 w428 w471 _ _]
          tunnel: w333 -> [_ _ _ _ w470 _ _]
          frame "Init", Default {
            # "1125?\nCari says 1050 \nBut 1050 too slow...\n1170? No\n870 for 2pt basket?\nNo. 940!\nNo, drop to 935"
            # "IS THIS EVEN NECESSARY?\n\n(no.)"
            # "SKIP AIMING\nGO STRAIGHT TO FIRE"
            # "Need input from dashboard"
            # "1: BASKET SELECTOR\n2: POSITION SELECTOR\n3: SHOOTER DELAY\n4: MOTOR SPEED"
            # "Constants NEED TO BE SET"
            # "This tells you the driver position\nand alliance color"
            # "This gives you the eight Driver Station\ndigital switch settings"
            # "This gives you the four\nDriver Station sliders or\nanalog voltages"
            n182 = call <vilib>:"WPI_DriverStationGet Alliance Info.vi"() -> ()  [unwired: 12 out]
            n183 = call <vilib>:"WPI_DriverStationGet Digital Input.vi"() -> ("Driver Station Digital Input (1-8)"=w377:bool[])  [unwired: 11 out]
            n184 = call <vilib>:"WPI_DriverStationGet Analog Input.vi"() -> ("Analog 4 (V)"=w348:dbl, "Analog 3 (V)"=w354:dbl, "Analog 2 (V)"=w355:dbl, "Analog 1 (V)"=w367:dbl)  [unwired: 8 out]
            n185 = global write "Robot Global Data.vi" "UseLauncherGyro"(TRUE) -> ()
            n186 = global write "Robot Global Data.vi" "UseRobotGyro"(TRUE) -> ()
            n187 = global write "Robot Global Data.vi" "Autonomous"(TRUE ("Autonomous")) -> ()
            n188 = global write "Robot Global Data.vi" "EnableAim"(FALSE) -> ()
            n189 = global write "Robot Global Data.vi" "Brake"(TRUE) -> ()
            n190 = Subtract(x=w348, y=2.5) -> (x-y=w346:dbl)
            n191 = Multiply(x=w346, y=40.0) -> (x*y=w343:dbl)
            n192 = global read "Robot Global Data.vi" "KeyRPM"() -> (w342:dbl)
            n193 = Greater?(x=w355, y=1.5) -> (0:w359:bool)
            n194 = Greater?(x=w367, y=1.5) -> (0:w371:bool)
            n195 = Greater?(x=w355, y=2.5) -> (0:w360:bool)
            n196 = Greater?(x=w355, y=3.5) -> (0:w361:bool)
            n197 = Greater?(x=w367, y=2.5) -> (0:w372:bool)
            n198 = Greater?(x=w367, y=3.5) -> (0:w373:bool)
            n199 = Add(x=w343, y=w342) -> (x+y=w344:dbl)
            n200 = Boolean To (0,1)(Boolean=w361) -> (0, 1=w356:i16)
            n201 = Boolean To (0,1)(Boolean=w373) -> (0, 1=w368:i16)
            n202 = Boolean To (0,1)(Boolean=w360) -> (0, 1=w357:i16)
            n203 = Boolean To (0,1)(Boolean=w372) -> (0, 1=w369:i16)
            n204 = Boolean To (0,1)(Boolean=w359) -> (0, 1=w358:i16)
            n205 = Index Array(array=w377) -> ()  [unwired: 8 in, 8 out]
            n206 = Boolean To (0,1)(Boolean=w371) -> (0, 1=w370:i16)
            n207 = global write "Robot Global Data.vi" "Set RPM"(w344) -> ()
            n208 = Compound Arithmetic op=ADD(w358, w357, w356) -> (w351:i16)
            n209 = Compound Arithmetic op=ADD(w370, w369, w368) -> (w341:i16)
            n210 = case shown="1, 3, Default" w351 {
              tunnel: [12.716666666666667 12.0] -> w352
              frame 1, 3, Default {
              }
              frame 2 {
              }
            }
            n211 = global write "Robot Global Data.vi" "SelectedIndex"(w341) -> ()
            n212 = global write "Robot Global Data.vi" "TargetDistance"(w352) -> ()
          }
          frame "Drive" {
            # "SKIPPED"
            n213 = while {
              shift-right: [w386] -> _
              shift-left: StateMachineType."Init" ("Enum") -> [w387]
              tunnel: [w384] -> w381
              tunnel: w380 -> [w383]
              stop <- w385 stop-if-true
              n214 = case shown="\"Start\"" w387 {
                selector: w387 -> [_ _ _ _ w398]
                tunnel: [StateMachineType."Idle" ("Enum") StateMachineType."Start" ("Enum") StateMachineType."Do" ("Enum") StateMachineType."Stop" ("Enum") w398] -> w386
                tunnel: [_ _ _ _ TRUE] -> w385
                tunnel: [_ _ _ _ AutonomousType."Fire" ("Enum")] -> w384
                tunnel: w383 -> [_ _ _ _ _]
                frame "Init", Default {
                }
                frame "Idle" {
                }
                frame "Start" {
                  w390 = 0.7 ("TankDriveLeft")
                  n215 = global write "Robot Global Data.vi" "TankDriveRight"(w390) -> ()
                  n216 = global write "Robot Global Data.vi" "TankDriveLeft"(w390) -> ()
                  n217 = Wait (ms)(milliseconds to wait=u32 1500) -> ()  [unwired: 1 out]
                }
                frame "Do" {
                  w393 = 0.35 ("TankDriveLeft")
                  n218 = global write "Robot Global Data.vi" "TankDriveRight"(w393) -> ()
                  n219 = global write "Robot Global Data.vi" "TankDriveLeft"(w393) -> ()
                  n220 = Wait (ms)(milliseconds to wait=u32 2500) -> ()  [unwired: 1 out]
                }
                frame "Stop" {
                  w396 = 0.0 ("TankDriveLeft")
                  n221 = global write "Robot Global Data.vi" "TankDriveRight"(w396) -> ()
                  n222 = global write "Robot Global Data.vi" "TankDriveLeft"(w396) -> ()
                }
              }
            }
          }
          frame "ManualAim" {
            # "SKIPPED"
            n223 = while {
              shift-right: [w406] -> _
              shift-left: StateMachineType."Init" ("Enum") -> [w407]
              tunnel: [w404] -> w401
              tunnel: w400 -> [w403]
              stop <- w405 stop-if-true
              n224 = case shown="\"Do\"" w407 {
                selector: w407 -> [_ w414 w426]
                tunnel: [StateMachineType."Do" ("Enum") w413 w426] -> w406
                tunnel: [_ _ TRUE] -> w405
                tunnel: [_ _ AutonomousType."AutoAim" ("Enum")] -> w404
                tunnel: w403 -> [_ w409 _]
                frame "Init", Default {
                }
                frame "Do" {
                  n225 = case shown="0, Default" w409 {
                    tunnel: [10.0 0.0 -10.0] -> w410
                    frame 0, Default {
                    }
                    frame 1 {
                      (unwired) 0.0
                      (unwired) 0.0
                    }
                    frame 2 {
                      (unwired) 2.11667
                      (unwired) 250.4
                    }
                  }
                  n226 = global read "Robot Global Data.vi" "LauncherGyro"() -> (w418:dbl)
                  n227 = Subtract(x=w410, y=w418) -> (x-y=w417:dbl)
                  n228 = call-poly <vilib>:"PID.vi"("output range"=cluster{"output high":dbl, "output low":dbl} {"output high"=1.0, "output low"=-1.0}, "PID gains"=T13 {"proportional gain (Kc)"=0.0016, "integral time (Ti, min)"=0.01, "derivative time (Td, min)"=0.0}, "process variable"=w418, "setpoint"=w410) -> ("output"=w419:dbl)  [unwired: 6 in, 1 out]
                  n229 = Less?(x=w417, y=1e-05) -> (x < y?=w415:bool)
                  n230 = global write "Robot Global Data.vi" "LauncherSteer"(w419) -> ()
                  n231 = Select(t=StateMachineType."Stop", s=w415, f=w414) -> (s? t:f=w413:T12)
                }
                frame "Stop" {
                  n232 = global write "Robot Global Data.vi" "LauncherSteer"(0.0 ("LauncherSteer")) -> ()
                }
              }
            }
          }
          frame "AutoAim" {
            # "SKIPPED"
            n233 = while {
              shift-right: [w434] -> _
              shift-left: StateMachineType."Init" ("Enum") -> [w435]
              tunnel: [w431] -> w429
              i -> [w432]
              stop <- w433 stop-if-true
              n234 = case shown="\"Do\"" w435 {
                selector: w435 -> [_ w447 w468]
                tunnel: [StateMachineType."Do" ("Enum") w446 w468] -> w434
                tunnel: [_ _ TRUE] -> w433
                tunnel: w432 -> [_ _ _]
                tunnel: [_ _ AutonomousType."Fire" ("Enum")] -> w431
                frame "Init", Default {
                  n235 = Wait (ms)(milliseconds to wait=u32 10) -> ()  [unwired: 1 out]
                  n236 = global write "Robot Global Data.vi" "EnableAim"(TRUE ("Enable Vision")) -> ()
                  n237 = global write "Robot Global Data.vi" "AutoCenter"(TRUE ("AutoCenter")) -> ()
                }
                frame "Do" {
                  n238 = disable-structure shown="Disabled" {
                    disable-tunnel: [w450 _] -> _
                    frame Disabled {
                      # "OFFSET"
                      n239 = global read "Robot Global Data.vi" "Target Info Legacy"() -> (w464:T14)
                      n240 = global read "Robot Global Data.vi" "SelectedIndex"() -> (w463:dbl)
                      n241 = Index Array(array=w464, index=w463) -> (element=w462:T15)
                      n242 = Unbundle By Name(w462) -> ("Position"=w461:cluster{"X":dbl, "Y":dbl})
                      n243 = Unbundle By Name(w461) -> ("Y"=w460:dbl)
                      n244 = Add(x=w460, y=0.0) -> (x+y=w448:dbl)
                      n245 = Greater?(x=w448, y=0.01) -> (0:w452:bool)
                      n246 = Less?(x=w448, y=-0.01) -> (x < y?=w451:bool)
                      n247 = Select(t=-0.1, s=w452, f=0.0) -> (s? t:f=w455:dbl)
                      n248 = Select(t=0.1, s=w451, f=w455) -> (s? t:f=w453:dbl)
                      n249 = Or(x=w451, y=w452) -> (x .or. y?=w450:bool)
                      n250 = global write "Robot Global Data.vi" "LauncherSteer"(w453) -> ()
                    }
                    frame Enabled {
                    }
                  }
                  n251 = global read "Robot Global Data.vi" "LauncherSteer"() -> (w443:dbl)
                  n252 = Absolute Value(x=w443) -> (abs(x)=w440:dbl)
                  n253 = Greater?(x=w440, y=0.01) -> (0:w441:bool)
                  n254 = Wait (ms)(milliseconds to wait=u32 10) -> ()  [unwired: 1 out]
                  n255 = Select(t=w447, s=w441, f=StateMachineType."Stop") -> (s? t:f=w446:T12)
                }
                frame "Stop" {
                  n256 = global write "Robot Global Data.vi" "AutoCenter"(FALSE ("AutoCenter")) -> ()
                  n257 = global write "Robot Global Data.vi" "EnableAim"(FALSE ("Enable Vision")) -> ()
                }
              }
            }
          }
          frame "Fire" {
            # "SKIPPING DRIVE & TIP RAMP"
            n258 = while {
              shift-right: [w479] -> _
              shift-left: StateMachineType."Init" ("Enum") -> [w480]
              tunnel: [w477] -> w472
              shift-right: [w476] -> _
              shift-left: _ -> [w475]
              tunnel: w470 -> [w474]
              stop <- w478 stop-if-true
              n259 = case shown="\"Do\"" w480 {
                selector: w480 -> [_ w487 _ w510 _]
                tunnel: [StateMachineType."Idle" ("Enum") w488 StateMachineType."Do" ("Enum") w509 w533] -> w479
                tunnel: [_ _ _ _ TRUE] -> w478
                tunnel: [_ _ _ _ w534] -> w477
                tunnel: [_ _ _ w512 _] -> w476
                tunnel: w475 -> [_ _ _ w511 _]
                tunnel: w474 -> [w482 _ _ _ _]
                frame "Init", Default {
                  n260 = Multiply(x=w482, y=1000.0) -> (x*y=w483:dbl)
                  n261 = global write "Robot Global Data.vi" "RunLauncher"(TRUE) -> ()
                  n262 = Wait (ms)(milliseconds to wait=w483) -> ()  [unwired: 1 out]
                }
                frame "Idle" {
                  # "TRUE: COMPARE SPEED\nFALSE: JUST WAIT 2 SECONDS"
                  n263 = case shown="False" FALSE {
                    tunnel: [StateMachineType."Start" ("Enum") w494] -> w488
                    tunnel: w487 -> [_ w492]
                    frame False {
                      n264 = global read "Robot Global Data.vi" "UpCloseRPMReverse"() -> (w489:dbl)
                      n265 = global write "Robot Global Data.vi" "Set RPM"(w489) -> ()
                      n266 = Wait (ms)(milliseconds to wait=u32 2000) -> ()  [unwired: 1 out]
                    }
                    frame True {
                      n267 = global read "Robot Global Data.vi" "LauncherSpeed"() -> (w499:dbl)
                      n268 = global read "Robot Global Data.vi" "Set RPM"() -> (w498:dbl)
                      n269 = Subtract(x=w499, y=w498) -> (x-y=w497:dbl)
                      n270 = Wait (ms)(milliseconds to wait=u32 10) -> ()  [unwired: 1 out]
                      n271 = Absolute Value(x=w497) -> (abs(x)=w495:dbl)
                      n272 = Less?(x=w495, y=50.0) -> (x < y?=w493:bool)
                      n273 = Select(t=StateMachineType."Start" ("Enum"), s=w493, f=w492) -> (s? t:f=w494:T12)
                    }
                  }
                }
                frame "Start" {
                  # "IN PERIODIC TASKS CREATE A BOOLEAN\nCONFIRMING THAT LAUNCHER IS UP TO SPEED"
                  # "MAKE FOR LOOP"
                  n274 = global read "Robot Global Data.vi" "UpCloseRPMReverse"() -> (w502:dbl)
                  n275 = local read "LaunchCounter 3"() -> (w505:i32)
                  n276 = global write "Robot Global Data.vi" "Ball Collector"(TRUE) -> ()
                  n277 = global write "Robot Global Data.vi" "Set RPM"(w502) -> ()
                  n278 = global write "Robot Global Data.vi" "Fire"(TRUE) -> ()
                  n279 = Increment(x=w505) -> (x+1=→"LaunchCounter 3":i32)
                }
                frame "Do" {
                  # "T: WAIT FOR SPEED DROP\nF: WAIT FOR 8 SECONDS"
                  # "This might be changed to just \"Wait for some set amount of time then move on\""
                  n280 = case shown="True" FALSE {
                    tunnel: [w516 w526] -> w512
                    tunnel: w511 -> [w516 w525]
                    tunnel: w510 -> [_ w520]
                    tunnel: [StateMachineType."Stop" ("t") w518] -> w509
                    frame False {
                      n281 = global read "Robot Global Data.vi" "UpCloseRPMReverse"() -> (w513:dbl)
                      n282 = global write "Robot Global Data.vi" "Set RPM"(w513) -> ()
                      n283 = Wait (ms)(milliseconds to wait=u32 8000) -> ()  [unwired: 1 out]
                    }
                    frame True {
                      n284 = global read "Robot Global Data.vi" "LauncherSpeed"() -> (w526:dbl)
                      n285 = Subtract(x=w526, y=w525) -> (x-y=w524:dbl)
                      n286 = Absolute Value(x=w524) -> (abs(x)=w522:dbl)
                      n287 = Greater?(x=w522, y=50.0) -> (0:w519:bool)
                      n288 = Select(t=StateMachineType."Stop", s=w519, f=w520) -> (s? t:f=w518:T12)
                      n289 = Wait (ms)(milliseconds to wait=u32 10) -> ()  [unwired: 1 out]
                    }
                  }
                }
                frame "Stop" {
                  # "T: WAIT FOR 2 BALLS LAUNCHED\nF: JUST STOP"
                  # "# OF BALLS IN COLLECTOR"
                  # "SKIPPING DRIVE"
                  n290 = local read "LaunchCounter 3"() -> (w536:i32)
                  n291 = global write "Robot Global Data.vi" "Ball Collector"(FALSE) -> ()
                  n292 = global write "Robot Global Data.vi" "Fire"(FALSE) -> ()
                  n293 = Select(t=2, s=FALSE, f=0 ("y")) -> (s? t:f=w527:i32)
                  n294 = Greater Or Equal?(x=w536, y=w527) -> (x >= y?=w535:bool)
                  n295 = case shown="False" w535 {
                    tunnel: [_ AutonomousType."Stop" ("Enum")] -> w534
                    tunnel: [StateMachineType."Idle" ("Enum") StateMachineType."Stop" ("Enum")] -> w533
                    frame False {
                    }
                    frame True {
                      # "SKIPPING DRIVE & TIP RAMP"
                      n296 = global write "Robot Global Data.vi" "RunLauncher"(FALSE) -> ()
                    }
                  }
                }
              }
            }
          }
          frame "Tip Ramp" {
            # "SKIPPED"
            n297 = while {
              shift-right: [w546] -> _
              shift-left: StateMachineType."Init" ("Enum") -> [w547]
              tunnel: [w544] -> w542
              stop <- w545 stop-if-true
              n298 = case shown="\"Idle\"" w547 {
                selector: w547 -> [_ w556 _ _ w568]
                tunnel: [StateMachineType."Idle" ("Enum") w555 StateMachineType."Do" ("Enum") StateMachineType."Stop" ("t") w568] -> w546
                tunnel: [_ _ _ _ TRUE] -> w545
                tunnel: [_ _ _ _ AutonomousType."Stop" ("Enum")] -> w544
                frame "Init", Default {
                }
                frame "Idle" {
                  w553 = 180.0 ("setpoint")
                  # "USE PID TO FACE RAMP"
                  n299 = global read "Robot Global Data.vi" "RobotGyro"() -> (w554:dbl)
                  n300 = Subtract(x=w554, y=w553) -> (x-y=w552:dbl)
                  n301 = call-poly <vilib>:"PID.vi"("output range"=cluster{"output high":dbl, "output low":dbl} {"output high"=1.0, "output low"=-1.0}, "PID gains"=T13 {"proportional gain (Kc)"=0.0016, "integral time (Ti, min)"=0.01, "derivative time (Td, min)"=0.0}, "process variable"=w554, "setpoint"=w553) -> ("output"=w560:dbl)  [unwired: 6 in, 1 out]
                  n302 = Absolute Value(x=w552) -> (abs(x)=w551:dbl)
                  n303 = Negate(x=w560) -> (-x=w559:dbl)
                  n304 = global write "Robot Global Data.vi" "TankDriveRight"(w559) -> ()
                  n305 = global write "Robot Global Data.vi" "TankDriveLeft"(w560) -> ()
                  n306 = Less?(x=w551, y=1.0) -> (x < y?=w549:bool)
                  n307 = Select(t=StateMachineType."Start" ("Enum"), s=w549, f=w556) -> (s? t:f=w555:T12)
                }
                frame "Start" {
                  n308 = global write "Robot Global Data.vi" "ArmActuate"(TRUE ("Arm")) -> ()
                }
                frame "Do" {
                  n309 = Wait (ms)(milliseconds to wait=u32 1000) -> ()  [unwired: 1 out]
                }
                frame "Stop" {
                  n310 = global write "Robot Global Data.vi" "ArmActuate"(FALSE) -> ()
                }
              }
            }
          }
          frame "Stop" {
            # "YAY DONE"
            n311 = global write "Robot Global Data.vi" "Autonomous"(FALSE) -> ()
            n312 = global write "Robot Global Data.vi" "UseLauncherGyro"(FALSE) -> ()
            n313 = global write "Robot Global Data.vi" "UseRobotGyro"(FALSE) -> ()
            n314 = Wait (ms)(milliseconds to wait=u32 100) -> ()  [unwired: 1 out]
          }
        }
      }
      n315 = while {
        shift-right: [w576] -> _
        shift-left: StateMachineType."Init" ("Enum") -> [w577]
        stop <- w575 stop-if-true
        n316 = case shown="\"Init\", Default" w577 {
          selector: w577 -> [w579 _ _ _ w591]
          tunnel: [w580 StateMachineType."Start" ("Enum") StateMachineType."Do" ("Enum") StateMachineType."Stop" ("Enum") w591] -> w576
          tunnel: [_ _ _ _ TRUE] -> w575
          frame "Init", Default {
            n317 = global read "Robot Global Data.vi" "Autonomous"() -> (w578:bool)
            n318 = Wait (ms)(milliseconds to wait=u32 1) -> ()  [unwired: 1 out]
            n319 = Select(t=StateMachineType."Idle" ("Enum"), s=w578, f=w579) -> (s? t:f=w580:T12)
          }
          frame "Idle" {
            w583 = 0.7 ("TankDriveLeft")
            n320 = global write "Robot Global Data.vi" "TankDriveRight"(w583) -> ()
            n321 = global write "Robot Global Data.vi" "TankDriveLeft"(w583) -> ()
            n322 = Wait (ms)(milliseconds to wait=u32 1800) -> ()  [unwired: 1 out]
          }
          frame "Start" {
            w586 = 0.4 ("TankDriveLeft")
            n323 = global write "Robot Global Data.vi" "TankDriveRight"(w586) -> ()
            n324 = global write "Robot Global Data.vi" "TankDriveLeft"(w586) -> ()
            n325 = Wait (ms)(milliseconds to wait=u32 2500) -> ()  [unwired: 1 out]
          }
          frame "Do" {
            w589 = 0.0 ("TankDriveLeft")
            n326 = global write "Robot Global Data.vi" "TankDriveRight"(w589) -> ()
            n327 = global write "Robot Global Data.vi" "TankDriveLeft"(w589) -> ()
          }
          frame "Stop" {
          }
        }
      }
    }
    frame Disabled {
    }
  }
  n328 = disable-structure shown="Disabled" {
    frame Disabled {
      n329 = call <vilib>:"WPI_RobotDriveRefNum Registry Get.vi"("refnum name"="TankDrive") -> ("RobotDriveDevRef"=w594:T2)  [unwired: 1 in, 9 out]
      n330 = while {
        shift-right: [w601] -> _
        shift-left: w594 -> [w602]
        tunnel: AutoDriveType."Stop" ("Enum") -> [w599]
        tunnel: [w598] -> _
        stop <- FALSE stop-if-true
        # "Drive"
        n331 = case shown="\"Drive\"" w599 {
          selector: w599 -> [w605 w611 w618]
          tunnel: w602 -> [w608 w616 w624]
          tunnel: [w608 w615 w623] -> w601
          tunnel: [w604 w610 w619] -> w598
          tunnel: "AutoDrive" -> [w606 w609 w617]
          frame "DoNothing" {
            n332 = Equal?(x=w605, y=w606) -> (x = y?=w607:bool)
            n333 = Select(t=w605, s=w607, f=w606) -> (s? t:f=w604:T1)
          }
          frame "Stop", Default {
            n334 = Equal?(x=w611, y=w609) -> (x = y?=w612:bool)
            n335 = call <vilib>:"WPI_RobotDriveTankDrive.vi"("Right axis value"=0.0, "Left axis value"=0.0, "RobotDriveDevRef"=w616) -> ("RobotDriveDevRef"=w615:T2)  [unwired: 7 in, 1 out]
            n336 = Select(t=w611, s=w612, f=w609) -> (s? t:f=w610:T1)
          }
          frame "Drive" {
            n337 = Equal?(x=w618, y=w617) -> (x = y?=w620:bool)
            n338 = call <vilib>:"WPI_RobotDriveTankDrive.vi"("Right axis value"=1.0, "Left axis value"=1.0, "RobotDriveDevRef"=w624) -> ("RobotDriveDevRef"=w623:T2)  [unwired: 7 in, 1 out]
            n339 = Select(t=w618, s=w620, f=w617) -> (s? t:f=w619:T1)
          }
        }
        n340 = Wait (ms)(milliseconds to wait=u32 50) -> ()  [unwired: 1 out]
        n341 = Wait (ms)(milliseconds to wait=u32 50) -> ()  [unwired: 1 out]
      }
    }
    frame Enabled {
    }
  }
  n342 = disable-structure shown="Disabled" {
    frame Disabled {
      # "DANGER"
      # "DANGER"
      # "DANGER"
      # "DANGER"
      # "DANGER"
      # "DANGER"
      # "DANGER"
      # "DANGER"
      # "DANGER"
      # "Shooter Delay"
      n343 = while {
        shift-right: [w631] -> _
        shift-left: _ -> [w629]
        shift-right: [w628] -> _
        shift-left: AutonomousType."Init" -> [w632]
        shift-right: [w627] -> _
        shift-left: _ -> [w626]
        stop <- FALSE stop-if-true
        n344 = case shown="\"Fire\"" w632 {
          selector: w632 -> [_ _ _ _ _ _ w876]
          tunnel: [w637 w671 w700 _ _ _ _] -> w631
          tunnel: w629 -> [_ w671 w700 _ _ _ _]
          tunnel: [AutonomousType."Fire" ("Enum") w670 w699 w730 w776 w845 w876] -> w628
          tunnel: [w634 w669 w698 w729 w775 _ _] -> w627
          tunnel: w626 -> [_ w669 w698 w729 w775 _ _]
          frame "Init", Default {
            # "GO STRAIGHT TO DRIVE\nDANGEROUS"
            # "1: BASKET SELECTOR\n2. BRIDGE SELECTOR\n3: SHOOTER DELAY"
            # "Constants NEED TO BE SET"
            # "This tells you the driver position\nand alliance color"
            # "This gives you the eight Driver Station\ndigital switch settings"
            # "This gives you the four\nDriver Station sliders or\nanalog voltages"
            n345 = call <vilib>:"WPI_DriverStationGet Alliance Info.vi"() -> ()  [unwired: 12 out]
            n346 = call <vilib>:"WPI_DriverStationGet Digital Input.vi"() -> ("Driver Station Digital Input (1-8)"=w662:bool[])  [unwired: 11 out]
            n347 = call <vilib>:"WPI_DriverStationGet Analog Input.vi"() -> ("Analog 3 (V)"=w637:dbl, "Analog 2 (V)"=w638:dbl, "Analog 1 (V)"=w650:dbl)  [unwired: 9 out]
            n348 = Greater?(x=w638, y=1.5) -> (0:w642:bool)
            n349 = Greater?(x=w650, y=1.5) -> (0:w656:bool)
            n350 = Greater?(x=w638, y=2.5) -> (0:w643:bool)
            n351 = Greater?(x=w638, y=3.5) -> (0:w644:bool)
            n352 = Greater?(x=w650, y=2.5) -> (0:w657:bool)
            n353 = Greater?(x=w650, y=3.5) -> (0:w658:bool)
            n354 = Boolean To (0,1)(Boolean=w644) -> (0, 1=w639:i16)
            n355 = Boolean To (0,1)(Boolean=w658) -> (0, 1=w653:i16)
            n356 = Boolean To (0,1)(Boolean=w643) -> (0, 1=w640:i16)
            n357 = Boolean To (0,1)(Boolean=w657) -> (0, 1=w654:i16)
            n358 = Boolean To (0,1)(Boolean=w642) -> (0, 1=w641:i16)
            n359 = Index Array(array=w662) -> ()  [unwired: 8 in, 8 out]
            n360 = Boolean To (0,1)(Boolean=w656) -> (0, 1=w655:i16)
            n361 = global write "Robot Global Data.vi" "UseLauncherGyro"(TRUE) -> ()
            n362 = global write "Robot Global Data.vi" "UseRobotGyro"(TRUE) -> ()
            n363 = Compound Arithmetic op=ADD(w641, w640, w639) -> (w634:i16)
            n364 = Compound Arithmetic op=ADD(w655, w654, w653) -> (w652:i16)
            n365 = global write "Robot Global Data.vi" "Brake"(TRUE) -> ()
            n366 = case shown="3" w652 {
              tunnel: [BasketType."Left" ("Basket") BasketType."Bottom" ("Basket") BasketType."Right" ("Basket") BasketType."Top" ("Basket")] -> w651
              frame 0, Default {
              }
              frame 1 {
              }
              frame 2 {
              }
              frame 3 {
              }
            }
            n367 = case shown="1, 3, Default" w634 {
              tunnel: [0.0 0.0] -> w633
              frame 1, 3, Default {
              }
              frame 2 {
              }
            }
            n368 = global write "Robot Global Data.vi" "TargetDistance"(w633) -> ()
            n369 = global write "Robot Global Data.vi" "Basket"(w651) -> ()
          }
          frame "ManualAim" {
            n370 = while {
              shift-right: [w676] -> _
              shift-left: StateMachineType."Init" ("Enum") -> [w677]
              tunnel: [w674] -> w670
              tunnel: w669 -> [w673]
              stop <- w675 stop-if-true
              n371 = case shown="\"Init\", Default" w677 {
                selector: w677 -> [_ w684 w696]
                tunnel: [StateMachineType."Do" ("Enum") w683 w696] -> w676
                tunnel: [_ _ TRUE] -> w675
                tunnel: [_ _ AutonomousType."AutoAim" ("Enum")] -> w674
                tunnel: w673 -> [_ w679 _]
                frame "Init", Default {
                }
                frame "Do" {
                  n372 = case shown="0, Default" w679 {
                    tunnel: [10.0 0.0 -10.0] -> w680
                    frame 0, Default {
                    }
                    frame 1 {
                      (unwired) 0.0
                      (unwired) 0.0
                    }
                    frame 2 {
                      (unwired) 2.11667
                      (unwired) 250.4
                    }
                  }
                  n373 = global read "Robot Global Data.vi" "LauncherGyro"() -> (w688:dbl)
                  n374 = Subtract(x=w680, y=w688) -> (x-y=w687:dbl)
                  n375 = call-poly <vilib>:"PID.vi"("output range"=cluster{"output high":dbl, "output low":dbl} {"output high"=1.0, "output low"=-1.0}, "PID gains"=T13 {"proportional gain (Kc)"=0.0016, "integral time (Ti, min)"=0.01, "derivative time (Td, min)"=0.0}, "process variable"=w688, "setpoint"=w680) -> ("output"=w689:dbl)  [unwired: 6 in, 1 out]
                  n376 = Less?(x=w687, y=1e-05) -> (x < y?=w685:bool)
                  n377 = global write "Robot Global Data.vi" "LauncherSteer"(w689) -> ()
                  n378 = Select(t=StateMachineType."Stop", s=w685, f=w684) -> (s? t:f=w683:T12)
                }
                frame "Stop" {
                  n379 = global write "Robot Global Data.vi" "LauncherSteer"(0.0 ("LauncherSteer")) -> ()
                }
              }
            }
          }
          frame "AutoAim" {
            n380 = while {
              shift-right: [w706] -> _
              shift-left: StateMachineType."Init" ("Enum") -> [w707]
              tunnel: w700 -> [w703]
              tunnel: [w702] -> w699
              i -> [w704]
              stop <- w705 stop-if-true
              n381 = case shown="\"Init\", Default" w707 {
                selector: w707 -> [_ w722 w727]
                tunnel: [StateMachineType."Do" ("Enum") w721 w727] -> w706
                tunnel: [_ _ TRUE] -> w705
                tunnel: w704 -> [_ w719 _]
                tunnel: w703 -> [_ w710 _]
                tunnel: [_ _ AutonomousType."Fire" ("Enum")] -> w702
                frame "Init", Default {
                  n382 = global write "Robot Global Data.vi" "EnableAim"(TRUE ("Enable Vision")) -> ()
                }
                frame "Do" {
                  w715 = u32 100 ("milliseconds to wait")
                  # "MIN AIM TIME"
                  n383 = Increment(x=w719) -> (x+1=w714:i32)
                  n384 = To Double Precision Float(number=w715) -> (double precision float=w716:dbl)
                  n385 = To Double Precision Float(number=w714) -> (double precision float=w713:dbl)
                  n386 = Add(x=2.0, y=w710) -> (x+y=w712:dbl)
                  n387 = Divide(x=w712, y=w716) -> (x/y=w717:dbl)
                  n388 = Greater Or Equal?(x=w713, y=w717) -> (x >= y?=w718:bool)
                  n389 = case shown="True" w718 {
                    tunnel: w715 -> [_ w723]
                    frame False {
                    }
                    frame True {
                      n390 = Wait (ms)(milliseconds to wait=w723) -> ()  [unwired: 1 out]
                    }
                  }
                  n391 = Select(t=StateMachineType."Stop", s=w718, f=w722) -> (s? t:f=w721:T12)
                }
                frame "Stop" {
                  n392 = global write "Robot Global Data.vi" "EnableAim"(FALSE ("Enable Vision")) -> ()
                  n393 = Wait (ms)(milliseconds to wait=u32 1000) -> ()  [unwired: 1 out]
                }
              }
            }
          }
          frame "Fire" {
            n394 = while {
              shift-right: [w736] -> _
              shift-left: StateMachineType."Init" ("Enum") -> [w737]
              tunnel: [w734] -> w730
              shift-right: [w733] -> _
              shift-left: _ -> [w732]
              stop <- w735 stop-if-true
              n395 = case shown="\"Stop\"" w737 {
                selector: w737 -> [_ w740 _ w756 _]
                tunnel: [StateMachineType."Idle" ("Enum") w742 StateMachineType."Do" ("Enum") w754 w765] -> w736
                tunnel: [_ _ _ _ TRUE] -> w735
                tunnel: [_ _ _ _ w766] -> w734
                tunnel: [_ _ _ w762 _] -> w733
                tunnel: w732 -> [_ _ _ w761 _]
                frame "Init", Default {
                  n396 = global write "Robot Global Data.vi" "RunLauncher"(TRUE) -> ()
                }
                frame "Idle" {
                  n397 = global read "Robot Global Data.vi" "LauncherSpeed"() -> (w747:dbl)
                  n398 = global read "Robot Global Data.vi" "Set RPM"() -> (w746:dbl)
                  n399 = Subtract(x=w747, y=w746) -> (x-y=w745:dbl)
                  n400 = Absolute Value(x=w745) -> (abs(x)=w743:dbl)
                  n401 = Less?(x=w743, y=50.0) -> (x < y?=w741:bool)
                  n402 = Wait (ms)(milliseconds to wait=u32 10) -> ()  [unwired: 1 out]
                  n403 = Select(t=StateMachineType."Start" ("Enum"), s=w741, f=w740) -> (s? t:f=w742:T12)
                }
                frame "Start" {
                  # "IN PERIODIC TASKS CREATE A BOOLEAN\nCONFIRMING THAT LAUNCHER IS UP TO SPEED"
                  # "MAKE FOR LOOP"
                  n404 = local read "LaunchCounter 2"() -> (w751:i32)
                  n405 = global write "Robot Global Data.vi" "Ball Collector"(TRUE) -> ()
                  n406 = Increment(x=w751) -> (x+1=→"LaunchCounter 2":i32)
                }
                frame "Do" {
                  n407 = global read "Robot Global Data.vi" "LauncherSpeed"() -> (w762:dbl)
                  n408 = Subtract(x=w762, y=w761) -> (x-y=w760:dbl)
                  n409 = Absolute Value(x=w760) -> (abs(x)=w758:dbl)
                  n410 = Greater?(x=w758, y=50.0) -> (0:w755:bool)
                  n411 = Select(t=StateMachineType."Stop", s=w755, f=w756) -> (s? t:f=w754:T12)
                  n412 = Wait (ms)(milliseconds to wait=u32 10) -> ()  [unwired: 1 out]
                }
                frame "Stop" {
                  n413 = local read "LaunchCounter 2"() -> (w769:i32)
                  n414 = global write "Robot Global Data.vi" "Ball Collector"(FALSE) -> ()
                  n415 = Greater Or Equal?(x=w769, y=3) -> (x >= y?=w767:bool)
                  n416 = case shown="True" w767 {
                    tunnel: [_ AutonomousType."Drive" ("Enum")] -> w766
                    tunnel: [StateMachineType."Idle" ("Enum") StateMachineType."Stop" ("Enum")] -> w765
                    frame False {
                    }
                    frame True {
                      n417 = global write "Robot Global Data.vi" "RunLauncher"(FALSE) -> ()
                    }
                  }
                }
              }
            }
          }
          frame "Drive" {
            n418 = while {
              shift-right: [w785] -> _
              shift-left: StateMachineType."Init" ("Enum") -> [w786]
              tunnel: [w783] -> w776
              shift-right: [w780] -> _
              shift-left: _ -> [w782]
              shift-right: [w778] -> _
              shift-left: _ -> [w781]
              tunnel: w775 -> [w779]
              stop <- w784 stop-if-true
              n419 = case shown="\"Idle\"" w786 {
                selector: w786 -> [_ w816 _ w835 w843]
                tunnel: [StateMachineType."Idle" ("Enum") w817 StateMachineType."Do" ("Enum") w834 w843] -> w785
                tunnel: [_ _ _ _ TRUE] -> w784
                tunnel: [_ _ _ _ AutonomousType."Tip Ramp" ("Enum")] -> w783
                tunnel: w782 -> [_ w814 w827 w832 _]
                tunnel: w781 -> [_ w813 _ _ _]
                tunnel: [w791 w814 w827 w832 _] -> w780
                tunnel: w779 -> [w808 _ _ _ _]
                tunnel: [w790 _ _ _ _] -> w778
                frame "Init", Default {
                  # "20.866666667-1.25"
                  # "BRIDGE Y COORDINATE"
                  # "DESIRED DISTANCE"
                  # "BRIDGE X COORDINATE"
                  # "DESIRED ANGLE"
                  n420 = global read "Robot Global Data.vi" "LauncherGyro"() -> (w787:dbl)
                  n421 = global read "Robot Global Data.vi" "TargetDistance"() -> (w788:dbl)
                  n422 = case shown="1, Default" w808 {
                    tunnel: [7.05 0.0 -7.05] -> w789
                    frame 1, Default {
                    }
                    frame 2 {
                    }
                    frame 3 {
                    }
                  }
                  n423 = Sine & Cosine(0:w787) -> (1:w801:dbl, 2:w800:dbl)
                  n424 = Multiply(x=w800, y=w788) -> (x*y=w806:dbl)
                  n425 = Multiply(x=w801, y=w788) -> (x*y=w807:dbl)
                  n426 = Add(x=w789, y=w807) -> (x+y=w798:dbl)
                  n427 = Subtract(x=19.616666666666667, y=w806) -> (x-y=w799:dbl)
                  n428 = Square(x=w799) -> (x^2=w804:dbl)
                  n429 = Square(x=w798) -> (x^2=w803:dbl)
                  n430 = Add(x=w804, y=w803) -> (x+y=w802:dbl)
                  n431 = Square Root(x=w802) -> (sqrt(x)=w791:dbl)
                  n432 = Inverse Tangent (2 Input)(1:w798, 2:w799) -> (0:w796:dbl)
                  n433 = Add(x=1.5707963267948966, y=w796) -> (x+y=w794:dbl)
                  n434 = Divide(x=w794, y=3.141592653589793) -> (x/y=w793:dbl)
                  n435 = Multiply(x=180.0, y=w793) -> (x*y=w790:dbl)
                }
                frame "Idle" {
                  n436 = global read "Robot Global Data.vi" "RobotGyro"() -> (w822:dbl)
                  n437 = Subtract(x=w822, y=w813) -> (x-y=w821:dbl)
                  n438 = call-poly <vilib>:"PID.vi"("output range"=cluster{"output high":dbl, "output low":dbl} {"output high"=1.0, "output low"=-1.0}, "PID gains"=T13 {"proportional gain (Kc)"=0.0016, "integral time (Ti, min)"=0.01, "derivative time (Td, min)"=0.0}, "process variable"=w822) -> ("output"=w825:dbl)  [unwired: 7 in, 1 out]
                  n439 = Absolute Value(x=w821) -> (abs(x)=w820:dbl)
                  n440 = Negate(x=w825) -> (-x=w824:dbl)
                  n441 = global write "Robot Global Data.vi" "TankDriveRight"(w824) -> ()
                  n442 = global write "Robot Global Data.vi" "TankDriveLeft"(w825) -> ()
                  n443 = Less?(x=w820, y=0.1) -> (x < y?=w815:bool)
                  n444 = Select(t=StateMachineType."Start" ("Enum"), s=w815, f=w816) -> (s? t:f=w817:T12)
                }
                frame "Start" {
                  # "Start driving straight"
                  n445 = global write "Robot Global Data.vi" "ReadDriveEncoders"(TRUE) -> ()
                  n446 = global write "Robot Global Data.vi" "TankDriveLeft"(1.0 ("TankDriveLeft")) -> ()
                  n447 = global write "Robot Global Data.vi" "StraightDrive"(TRUE) -> ()
                }
                frame "Do" {
                  n448 = global read "Robot Global Data.vi" "DriveDistance"() -> (w837:dbl)
                  n449 = Greater?(x=w837, y=w832) -> (0:w833:bool)
                  n450 = case shown="True" w833 {
                    frame False {
                    }
                    frame True {
                      n451 = Wait (ms)(milliseconds to wait=u32 50) -> ()  [unwired: 1 out]
                    }
                  }
                  n452 = Select(t=StateMachineType."Stop", s=w833, f=w835) -> (s? t:f=w834:T12)
                }
                frame "Stop" {
                  n453 = global write "Robot Global Data.vi" "ReadDriveEncoders"(FALSE) -> ()
                  n454 = global write "Robot Global Data.vi" "TankDriveLeft"(0.0 ("TankDriveLeft")) -> ()
                  n455 = global write "Robot Global Data.vi" "StraightDrive"(FALSE) -> ()
                }
              }
            }
          }
          frame "Tip Ramp" {
            n456 = while {
              shift-right: [w849] -> _
              shift-left: StateMachineType."Init" ("Enum") -> [w850]
              tunnel: [w847] -> w845
              stop <- w848 stop-if-true
              n457 = case shown="\"Init\", Default" w850 {
                selector: w850 -> [_ w859 _ _ w871]
                tunnel: [StateMachineType."Idle" ("Enum") w858 StateMachineType."Do" ("Enum") StateMachineType."Stop" ("t") w871] -> w849
                tunnel: [_ _ _ _ TRUE] -> w848
                tunnel: [_ _ _ _ AutonomousType."Stop" ("Enum")] -> w847
                frame "Init", Default {
                }
                frame "Idle" {
                  w856 = 180.0 ("setpoint")
                  # "USE PID TO FACE RAMP"
                  n458 = global read "Robot Global Data.vi" "RobotGyro"() -> (w857:dbl)
                  n459 = Subtract(x=w857, y=w856) -> (x-y=w855:dbl)
                  n460 = call-poly <vilib>:"PID.vi"("output range"=cluster{"output high":dbl, "output low":dbl} {"output high"=1.0, "output low"=-1.0}, "PID gains"=T13 {"proportional gain (Kc)"=0.0016, "integral time (Ti, min)"=0.01, "derivative time (Td, min)"=0.0}, "process variable"=w857, "setpoint"=w856) -> ("output"=w863:dbl)  [unwired: 6 in, 1 out]
                  n461 = Absolute Value(x=w855) -> (abs(x)=w854:dbl)
                  n462 = Negate(x=w863) -> (-x=w862:dbl)
                  n463 = global write "Robot Global Data.vi" "TankDriveRight"(w862) -> ()
                  n464 = global write "Robot Global Data.vi" "TankDriveLeft"(w863) -> ()
                  n465 = Less?(x=w854, y=1.0) -> (x < y?=w852:bool)
                  n466 = Select(t=StateMachineType."Start" ("Enum"), s=w852, f=w859) -> (s? t:f=w858:T12)
                }
                frame "Start" {
                  n467 = global write "Robot Global Data.vi" "ArmActuate"(TRUE ("Arm")) -> ()
                }
                frame "Do" {
                  n468 = Wait (ms)(milliseconds to wait=u32 1000) -> ()  [unwired: 1 out]
                }
                frame "Stop" {
                  n469 = global write "Robot Global Data.vi" "ArmActuate"(FALSE) -> ()
                }
              }
            }
          }
          frame "Stop" {
            # "YAY DONE"
            n470 = global write "Robot Global Data.vi" "UseLauncherGyro"(FALSE) -> ()
            n471 = global write "Robot Global Data.vi" "UseRobotGyro"(FALSE) -> ()
            n472 = Wait (ms)(milliseconds to wait=u32 100) -> ()  [unwired: 1 out]
          }
        }
      }
    }
    frame Enabled {
    }
  }
